vi "Main Page.vi"(8 "error in (no error)":errorcluster, 11 "Node Ptr":T5 format="%.0x") -> (0 "error out":errorcluster)   [LabVIEW 2017, in "ALMA_10201-10401_O2SensorSim System Explorer.lvlib"]
uses:
  ALMA_10201-10401_O2SensorSim System Explorer.lvlib
  Engine/LambdaType.ctl
  <vilib>/NI Veristand/Custom Device API/Custom Device Item Ref.ctl
  Engine/Par.ctl
  <vilib>/Utility/sysdir.llb/System Directory Type.ctl
  Shared/Constants.vi
  <vilib>/NI Veristand/Custom Device API/Get Item Property (U32).vi
  <vilib>/NI Veristand/Custom Device API/Get Item Property (Boolean).vi
  <vilib>/NI Veristand/Custom Device API/Set Item Property (Boolean).vi
  <vilib>/NI Veristand/Custom Device API/Get Item Property (String).vi
  <userlib>/_OpenG.lib/comparison/comparison.llb/I32 Changed__ogtk.vi
  <userlib>/_OpenG.lib/comparison/comparison.llb/Variant Changed__ogtk.vi
  <vilib>/NI Veristand/Custom Device API/Set Item Property (String).vi
  <vilib>/NI Veristand/Custom Device API/Custom Device API.lvlib
  <vilib>/NI Veristand/Custom Device API/Set Item Property (U32).vi
  Shared/ALMA_10201-10401_O2SensorSim Shared.lvlib
panel:
  out "product.Num":u32
  out "vendor.Num":u32
  out "SLSC Module Name":string
  out "Version":string
  out "Board":string
  out "Module Number":u32
  out "Temperature [°C] VS Rs [W]":cluster{"Custom Temp":dbl[], "Custom Ohm":dbl[]}(graph)
  out "l VS IP [mA]":T1(graph)
  in  "Mode":u16(ring) items=["SLSC Mode", "ANALOG Mode"]
  out "RefArray":refnum<vi>[](array[refnum])
  in  "Processor":i32=-2
  in  "Period [ms]":i64=100
  in  "Manual":bool
  in  "Description":string
  in  "Name":string
  in  "ParamUpdate":bool=TRUE
  in  "par 3":T2={"Loop time"={"Period [ms]"=0, "Processor"=0}, "COM"={"COM IP"="0.0.0.0", "COM port"=1, "Local port"=0, "Next_IP 1"=0, "Next_IP 2"=0, "Next_IP 3"=0, "Next_IP 4"=0}, "O2Sensor1"={"Lambda"={"LSU4.2 Lambda"=[], "LSU4.2 Ip"=[], "LSU4.9 Lambda"=[], "LSU4.9 Ip"=[], "LZA03 Lambda"=[], "LZA03 Ip"=[], "LZA08 Lambda"=[], "LZA08 Ip"=[], "Custom Lambda"=[], "Custom Ip"=[]}, "Temp"={"LSU4.2 Temp"=[], "LSU4.2 Ohm"=[], "LSU4.9 Temp"=[], "LSU4.9 Ohm"=[], "LZA03 Temp"=[], "LZA03 Ohm"=[], "LZA08 Temp"=[], "LZA08 Ohm"=[], "Custom Temp"=[], "Custom Ohm"=[]}, "Lambda Type"=0, "PID"={"Ki"=0.0, "Kp"=0.0, "Kd"=0.0, "FeedFW"=0.0}}, "O2Sensor2"={"Lambda"={"LSU4.2 Lambda"=[], "LSU4.2 Ip"=[], "LSU4.9 Lambda"=[], "LSU4.9 Ip"=[], "LZA03 Lambda"=[], "LZA03 Ip"=[], "LZA08 Lambda"=[], "LZA08 Ip"=[], "Custom Lambda"=[], "Custom Ip"=[]}, "Temp"={"LSU4.2 Temp"=[], "LSU4.2 Ohm"=[], "LSU4.9 Temp"=[], "LSU4.9 Ohm"=[], "LZA03 Temp"=[], "LZA03 Ohm"=[], "LZA08 Temp"=[], "LZA08 Ohm"=[], "Custom Temp"=[], "Custom Ohm"=[]}, "Lambda Type"=0, "PID"={"Ki"=0.0, "Kp"=0.0, "Kd"=0.0, "FeedFW"=0.0}}, "O2Sensor3"={"Lambda"={"LSU4.2 Lambda"=[], "LSU4.2 Ip"=[], "LSU4.9 Lambda"=[], "LSU4.9 Ip"=[], "LZA03 Lambda"=[], "LZA03 Ip"=[], "LZA08 Lambda"=[], "LZA08 Ip"=[], "Custom Lambda"=[], "Custom Ip"=[]}, "Temp"={"LSU4.2 Temp"=[], "LSU4.2 Ohm"=[], "LSU4.9 Temp"=[], "LSU4.9 Ohm"=[], "LZA03 Temp"=[], "LZA03 Ohm"=[], "LZA08 Temp"=[], "LZA08 Ohm"=[], "Custom Temp"=[], "Custom Ohm"=[]}, "Lambda Type"=0, "PID"={"Ki"=0.0, "Kp"=0.0, "Kd"=0.0, "FeedFW"=0.0}}, "O2Sensor4"={"Lambda"={"LSU4.2 Lambda"=[], "LSU4.2 Ip"=[], "LSU4.9 Lambda"=[], "LSU4.9 Ip"=[], "LZA03 Lambda"=[], "LZA03 Ip"=[], "LZA08 Lambda"=[], "LZA08 Ip"=[], "Custom Lambda"=[], "Custom Ip"=[]}, "Temp"={"LSU4.2 Temp"=[], "LSU4.2 Ohm"=[], "LSU4.9 Temp"=[], "LSU4.9 Ohm"=[], "LZA03 Temp"=[], "LZA03 Ohm"=[], "LZA08 Temp"=[], "LZA08 Ohm"=[], "Custom Temp"=[], "Custom Ohm"=[]}, "Lambda Type"=0, "PID"={"Ki"=0.0, "Kp"=0.0, "Kd"=0.0, "FeedFW"=0.0}}, "#ch_choise"=enum."O2Sim_2ch", "Mode"=enum."SLSC Mode", "vendor.Num"=4141, "product.Num"=0} {"O2Sensor4"."Lambda Type" items=["LSU4.2", "LSU4.9", "LZA03", "LZA08", "Custom", "[mA]"]; "O2Sensor3"."Lambda Type" items=["LSU4.2", "LSU4.9", "LZA03", "LZA08", "Custom", "[mA]"]; "O2Sensor2"."Lambda Type" items=["LSU4.2", "LSU4.9", "LZA03", "LZA08", "Custom", "[mA]"]; "O2Sensor1"."Lambda Type" items=["LSU4.2", "LSU4.9", "LZA03", "LZA08", "Custom", "[mA]"]}
  in  "Tab Control 2":T4(tab)=enum."O2Sensor4"
  in  "Caratteristica LSU4.2":dbl[][](array[numeric])
  in  "Caratteristica Bosch":dbl[][](array[numeric])
  in  "Caratteristica LZA08":dbl[][](array[numeric])
  in  "Caratteristica LZA03":dbl[][](array[numeric])
  in  "Caratteristica Custom":dbl[][](array[numeric])
  in  "Caratteristica LSU4.2_temp":dbl[][](array[numeric])
  in  "Caratteristica Bosch_temp":dbl[][](array[numeric])
  in  "Caratteristica LZA03_temp":dbl[][](array[numeric])
  in  "Caratteristica LZA08_temp":dbl[][](array[numeric])
  in  "Caratteristica Custom_temp":dbl[][](array[numeric])
  in  "Lambda":string="Lambda"
  in  "Ip [mA]":string="Ip [mA]"
  in  "Temp [°]":string="Temp [°]"
  in  "R [Ohm]":string="R [Ohm]"
  in  "O2Sensor Type":T3 items=["LSU4.2", "LSU4.9", "LZA03", "LZA08", "Custom", "[mA]"]
  in  "PID.Kp_1":dbl
  in  "PID.Kd_1":dbl
  in  "PID.FeedFW_1":dbl
  in  "PID.Ki_1":dbl
  in  "Import":bool
  in  "Caratteristica Custom 2":dbl[][](array[numeric])
  in  "Caratteristica LZA03 2":dbl[][](array[numeric])
  in  "Caratteristica LZA08 2":dbl[][](array[numeric])
  in  "Caratteristica Bosch 2":dbl[][](array[numeric])
  in  "Caratteristica LSU4.2 2":dbl[][](array[numeric])
  in  "Caratteristica Custom_temp 2":dbl[][](array[numeric])
  in  "Caratteristica LZA08_temp 2":dbl[][](array[numeric])
  in  "Caratteristica LZA03_temp 2":dbl[][](array[numeric])
  in  "Caratteristica Bosch_temp 2":dbl[][](array[numeric])
  in  "Caratteristica LSU4.2_temp 2":dbl[][](array[numeric])
  in  "R [Ohm] 2":string="R [Ohm]"
  in  "Temp [°] 2":string="Temp [°]"
  in  "Ip [mA] 2":string="Ip [mA]"
  in  "Lambda 2":string="Lambda"
  in  "PID.Ki_2":dbl=0.005
  in  "PID.FeedFW_2":dbl
  in  "PID.Kd_2":dbl
  in  "PID.Kp_2":dbl=100.0
  in  "O2Sensor Type 2":T3 items=["LSU4.2", "LSU4.9", "LZA03", "LZA08", "Custom", "[mA]"]
  in  "Import 2":bool
  in  "Caratteristica Custom 3":dbl[][](array[numeric])
  in  "Caratteristica LZA03 3":dbl[][](array[numeric])
  in  "Caratteristica LZA08 3":dbl[][](array[numeric])
  in  "Caratteristica Bosch 3":dbl[][](array[numeric])
  in  "Caratteristica LSU4.2 3":dbl[][](array[numeric])
  in  "Caratteristica Custom_temp 3":dbl[][](array[numeric])
  in  "Caratteristica LZA08_temp 3":dbl[][](array[numeric])
  in  "Caratteristica LZA03_temp 3":dbl[][](array[numeric])
  in  "Caratteristica Bosch_temp 3":dbl[][](array[numeric])
  in  "Caratteristica LSU4.2_temp 3":dbl[][](array[numeric])
  in  "R [Ohm] 3":string="R [Ohm]"
  in  "Temp [°] 3":string="Temp [°]"
  in  "Ip [mA] 3":string="Ip [mA]"
  in  "Lambda 3":string="Lambda"
  in  "PID.Ki_3":dbl=0.005
  in  "PID.FeedFW_3":dbl
  in  "PID.Kd_3":dbl
  in  "PID.Kp_3":dbl=100.0
  in  "O2Sensor Type 3":T3 items=["LSU4.2", "LSU4.9", "LZA03", "LZA08", "Custom", "[mA]"]
  in  "Import 3":bool
  in  "Caratteristica LSU4.2 4":dbl[][](array[numeric])
  in  "Caratteristica Bosch 4":dbl[][](array[numeric])
  in  "Caratteristica LZA03 4":dbl[][](array[numeric])
  in  "Caratteristica LZA08 4":dbl[][](array[numeric])
  in  "Caratteristica Custom 4":dbl[][](array[numeric])
  in  "Caratteristica LSU4.2_temp 4":dbl[][](array[numeric])
  in  "Caratteristica Custom_temp 4":dbl[][](array[numeric])
  in  "Caratteristica LZA08_temp 4":dbl[][](array[numeric])
  in  "Caratteristica LZA03_temp 4":dbl[][](array[numeric])
  in  "Caratteristica Bosch_temp 4":dbl[][](array[numeric])
  in  "Temp [°] 4":string="Temp [°]"
  in  "Ip [mA] 4":string="Ip [mA]"
  in  "Lambda 4":string="Lambda"
  in  "PID.Ki_4":dbl=0.005
  in  "PID.Kd_4":dbl
  in  "PID.Kp_4":dbl=100.0
  in  "O2Sensor Type 4":T3 items=["LSU4.2", "LSU4.9", "LZA03", "LZA08", "Custom", "[mA]"]
  in  "Import 4":bool
  in  "PID.FeedFW_4":dbl
  in  "R [Ohm] 4":string="R [Ohm]"
  in  "Header":cluster{"Section Name":string}={"Section Name"="Custom Device Item Settings"}
  # "l VS IP [mA]_"
  # "Temperature [°C] VS Rs [W]_"
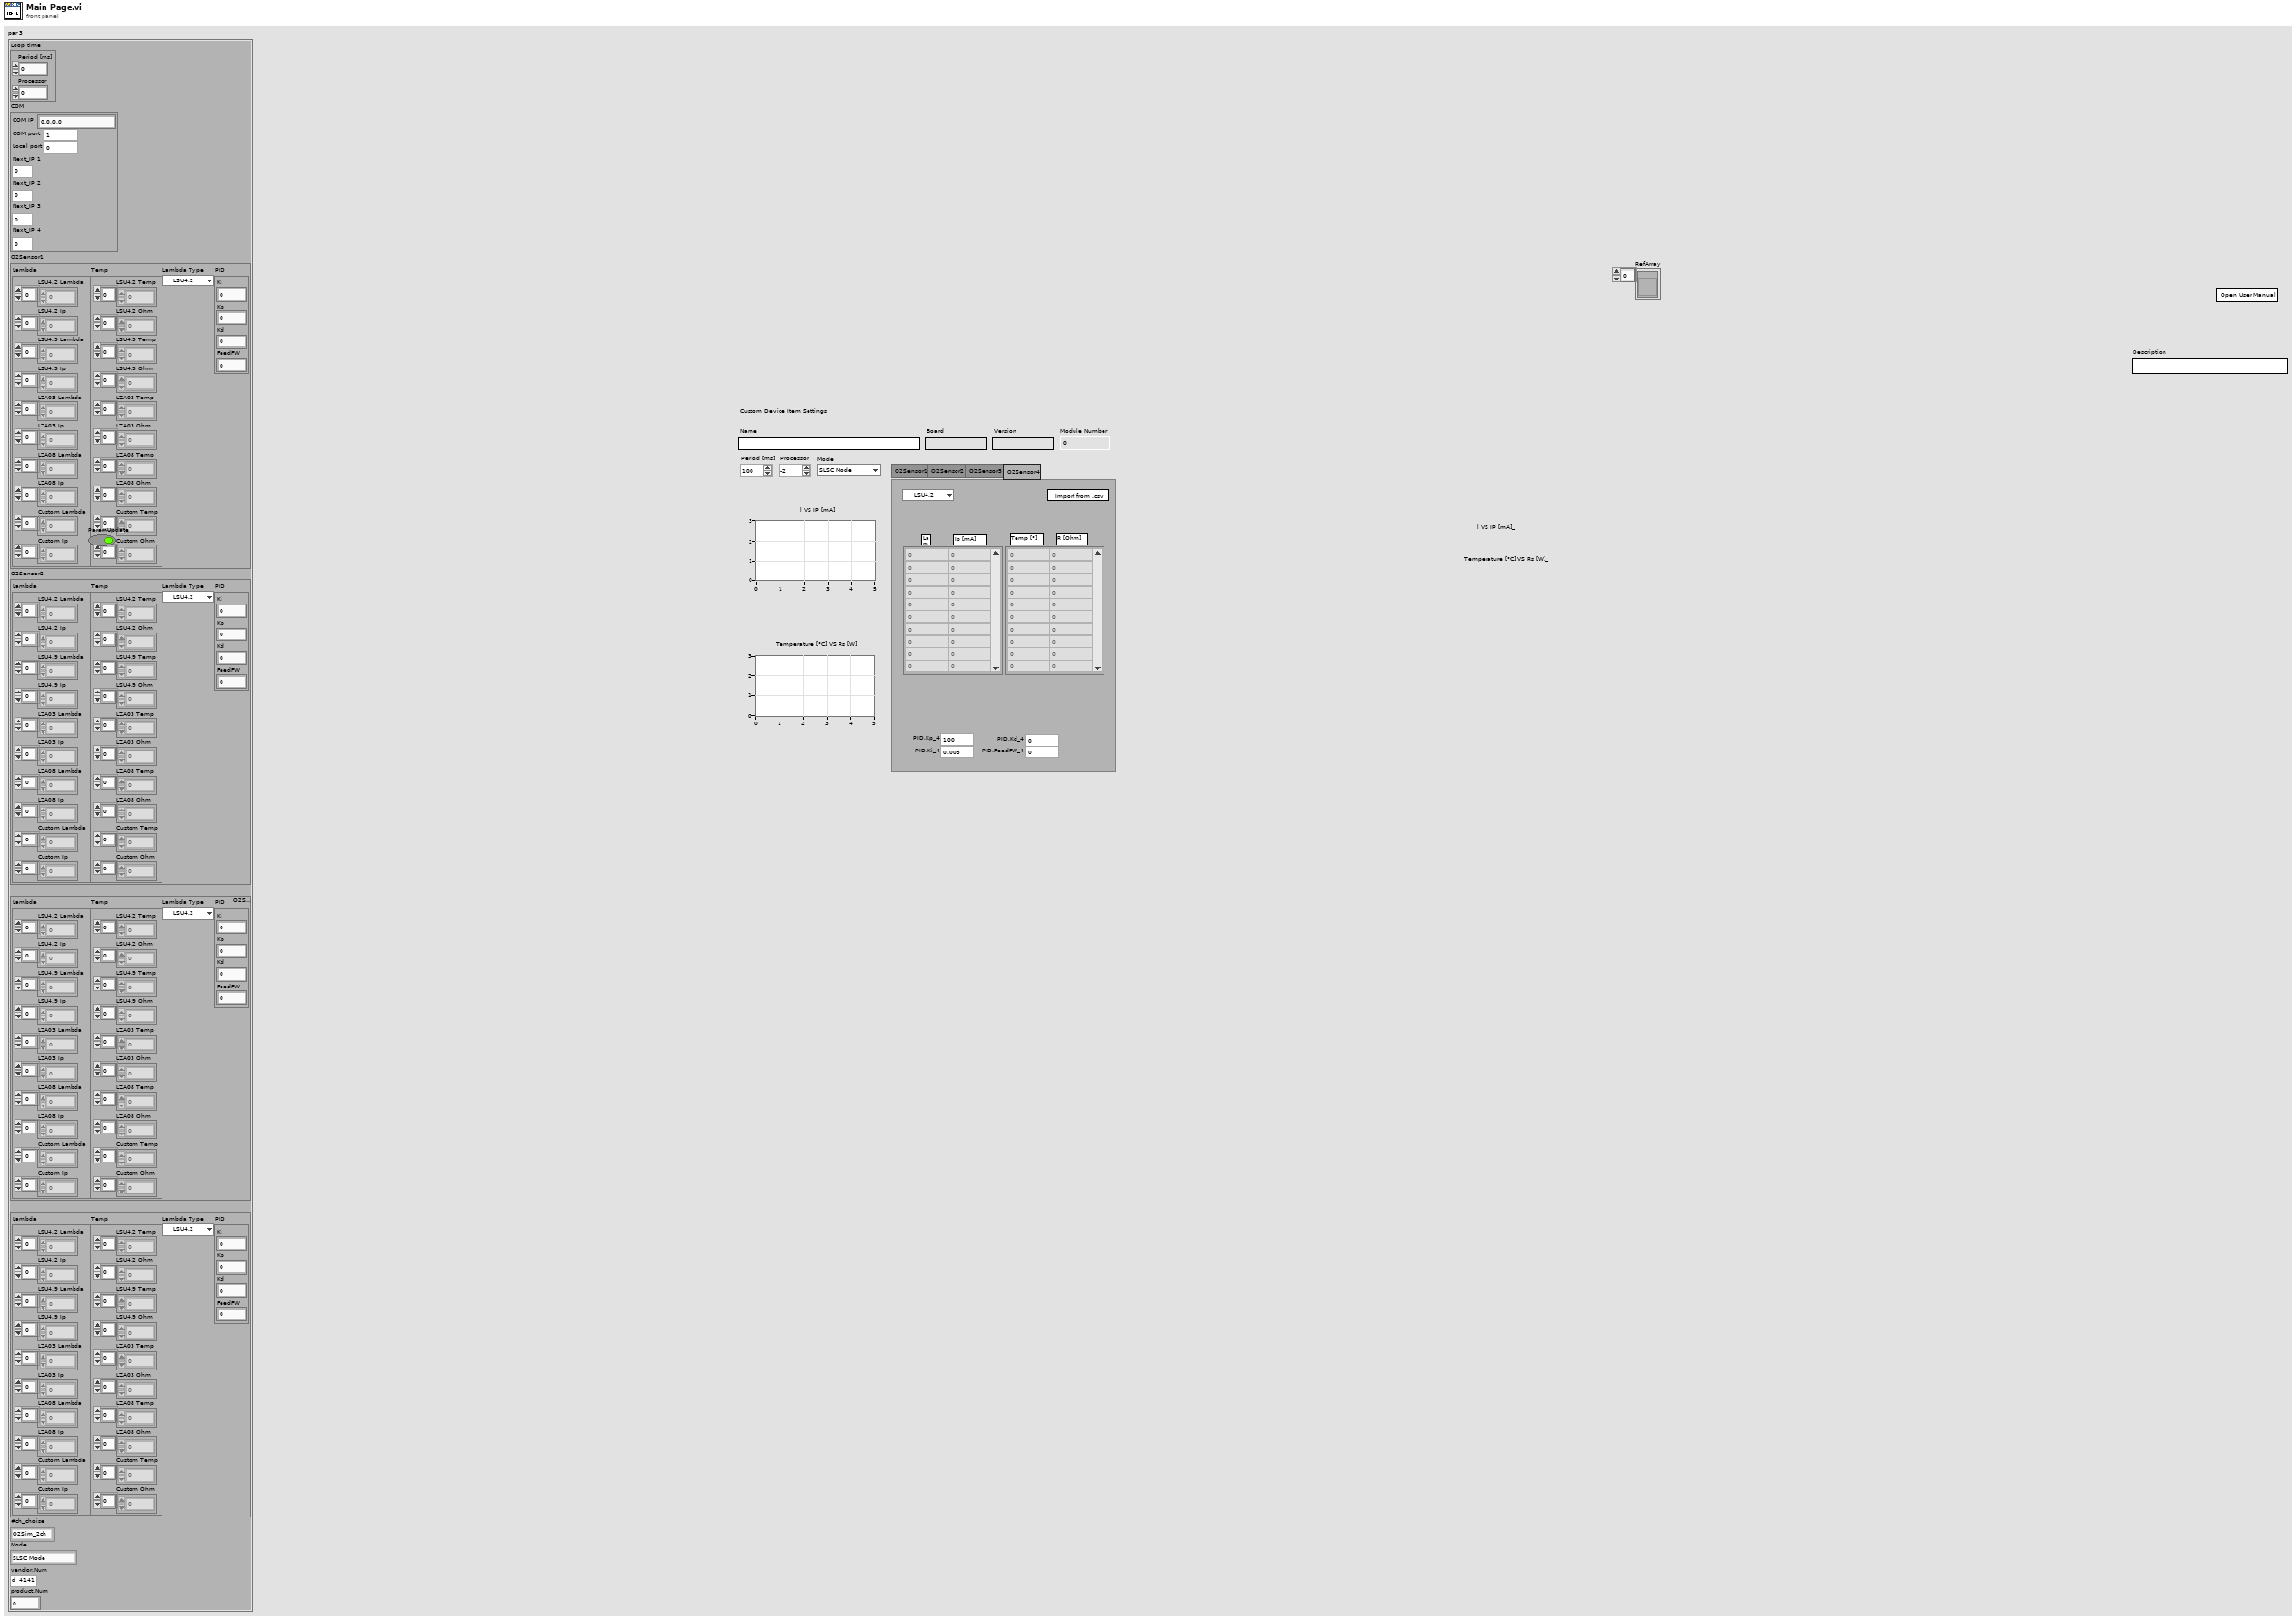
[diagram p1: front panel]
types:
  T1 = cluster{"Custom Lambda":dbl[], "Custom Ip":dbl[]}
  T2 = typedef "Par.ctl" = cluster{"Loop time":cluster{"Period [ms]":i64, "Processor":i32}, "COM":cluster{"COM IP":string, "COM port":u64, "Local port":u64, "Next_IP 1":u32, "Next_IP 2":u32, "Next_IP 3":u32, "Next_IP 4":u32}, "O2Sensor1":cluster{"Lambda":cluster{"LSU4.2 Lambda":dbl[], "LSU4.2 Ip":dbl[], "LSU4.9 Lambda":dbl[], "LSU4.9 Ip":dbl[], "LZA03 Lambda":dbl[], "LZA03 Ip":dbl[], "LZA08 Lambda":dbl[], "LZA08 Ip":dbl[], "Custom Lambda":dbl[], "Custom Ip":dbl[]}, "Temp":cluster{"LSU4.2 Temp":dbl[], "LSU4.2 Ohm":dbl[], "LSU4.9 Temp":dbl[], "LSU4.9 Ohm":dbl[], "LZA03 Temp":dbl[], "LZA03 Ohm":dbl[], "LZA08 Temp":dbl[], "LZA08 Ohm":dbl[], "Custom Temp":dbl[], "Custom Ohm":dbl[]}, "Lambda Type":T3, "PID":cluster{"Ki":dbl, "Kp":dbl, "Kd":dbl, "FeedFW":dbl}}, "O2Sensor2":cluster{"Lambda":cluster{"LSU4.2 Lambda":dbl[], "LSU4.2 Ip":dbl[], "LSU4.9 Lambda":dbl[], "LSU4.9 Ip":dbl[], "LZA03 Lambda":dbl[], "LZA03 Ip":dbl[], "LZA08 Lambda":dbl[], "LZA08 Ip":dbl[], "Custom Lambda":dbl[], "Custom Ip":dbl[]}, "Temp":cluster{"LSU4.2 Temp":dbl[], "LSU4.2 Ohm":dbl[], "LSU4.9 Temp":dbl[], "LSU4.9 Ohm":dbl[], "LZA03 Temp":dbl[], "LZA03 Ohm":dbl[], "LZA08 Temp":dbl[], "LZA08 Ohm":dbl[], "Custom Temp":dbl[], "Custom Ohm":dbl[]}, "Lambda Type":T3, "PID":cluster{"Ki":dbl, "Kp":dbl, "Kd":dbl, "FeedFW":dbl}}, "O2Sensor3":cluster{"Lambda":cluster{"LSU4.2 Lambda":dbl[], "LSU4.2 Ip":dbl[], "LSU4.9 Lambda":dbl[], "LSU4.9 Ip":dbl[], "LZA03 Lambda":dbl[], "LZA03 Ip":dbl[], "LZA08 Lambda":dbl[], "LZA08 Ip":dbl[], "Custom Lambda":dbl[], "Custom Ip":dbl[]}, "Temp":cluster{"LSU4.2 Temp":dbl[], "LSU4.2 Ohm":dbl[], "LSU4.9 Temp":dbl[], "LSU4.9 Ohm":dbl[], "LZA03 Temp":dbl[], "LZA03 Ohm":dbl[], "LZA08 Temp":dbl[], "LZA08 Ohm":dbl[], "Custom Temp":dbl[], "Custom Ohm":dbl[]}, "Lambda Type":T3, "PID":cluster{"Ki":dbl, "Kp":dbl, "Kd":dbl, "FeedFW":dbl}}, "O2Sensor4":cluster{"Lambda":cluster{"LSU4.2 Lambda":dbl[], "LSU4.2 Ip":dbl[], "LSU4.9 Lambda":dbl[], "LSU4.9 Ip":dbl[], "LZA03 Lambda":dbl[], "LZA03 Ip":dbl[], "LZA08 Lambda":dbl[], "LZA08 Ip":dbl[], "Custom Lambda":dbl[], "Custom Ip":dbl[]}, "Temp":cluster{"LSU4.2 Temp":dbl[], "LSU4.2 Ohm":dbl[], "LSU4.9 Temp":dbl[], "LSU4.9 Ohm":dbl[], "LZA03 Temp":dbl[], "LZA03 Ohm":dbl[], "LZA08 Temp":dbl[], "LZA08 Ohm":dbl[], "Custom Temp":dbl[], "Custom Ohm":dbl[]}, "Lambda Type":T3, "PID":cluster{"Ki":dbl, "Kp":dbl, "Kd":dbl, "FeedFW":dbl}}, "#ch_choise":enum16{"O2Sim_2ch", "O2Sim_4ch"}, "Mode":enum16{"SLSC Mode", "ANALOG Mode"}, "vendor.Num":u32, "product.Num":u32}
  T3 = typedef "LambdaType.ctl" = u16
  T4 = enum32{"O2Sensor1", "O2Sensor2", "O2Sensor3", "O2Sensor4"}
  T5 = typedef "Custom Device API.lvlib/Custom Device Item Ref.ctl" = u64
  T6 = typedef "Custom Device API.lvlib/Custom Device Item Info.ctl" = cluster{"Name":string, "Is Channel":bool, "GUID":string, "Is Waveform":bool}
  T7 = typedef "EDSjsonStructure.ctl" = cluster{"vendorNum":u32, "vendorName":string, "vendorPrefix":string, "productNum":u32, "productName":string, "capsVersion":string, "capsSpecVersion":u32, "capsSpecOldestCompatibleVersion":u32, "enums":T8[], "properties":T9[], "commands":T10[], "scales":T11[], "physicalChannels":T12[], "registerMap":cluster{"registers":T13[]}}
  T8 = typedef "enum.ctl" = cluster{"name":string, "description-en":string, "values":cluster{"name":string, "description-en":string, "value":i32}[]}
  T9 = typedef "property.ctl" = cluster{"name":string, "description-en":string, "documentation-en":string, "dataType":string, "bitfield":string, "access":string, "scale":string, "value":variant, "min":variant, "max":variant, "default value":variant}
  T10 = typedef "command.ctl" = cluster{"name":string, "description-en":string, "documentation-en":string, "startBitfield":string, "waitTimeInMs":i32, "doneBitfield":string, "doneInterrupt":string, "doneTimeoutInMs":i32, "value":variant}
  T11 = typedef "scale.ctl" = cluster{"name":string, "description-en":string, "m":dbl, "b":dbl, "forwardCoeffs":dbl[], "reverseCoeffs":dbl[], "coercion":string, "table":cluster{"scaled":dbl, "unscaled":dbl}[]}
  T12 = typedef "physicalChannel.ctl" = cluster{"name":string, "description-en":string, "commands":T10[], "properties":T9[]}
  T13 = typedef "register.ctl" = cluster{"name":string, "description-en":string, "access":string, "address":u32, "size":u32, "bitfields":cluster{"name":string, "description-en":string, "offset":u32, "size":u32, "signed":bool, "strobe":bool}[]}
  T14 = cluster{"Lambda":cluster{"LSU4.2 Lambda":dbl[], "LSU4.2 Ip":dbl[], "LSU4.9 Lambda":dbl[], "LSU4.9 Ip":dbl[], "LZA03 Lambda":dbl[], "LZA03 Ip":dbl[], "LZA08 Lambda":dbl[], "LZA08 Ip":dbl[], "Custom Lambda":dbl[], "Custom Ip":dbl[]}, "Temp":cluster{"LSU4.2 Temp":dbl[], "LSU4.2 Ohm":dbl[], "LSU4.9 Temp":dbl[], "LSU4.9 Ohm":dbl[], "LZA03 Temp":dbl[], "LZA03 Ohm":dbl[], "LZA08 Temp":dbl[], "LZA08 Ohm":dbl[], "Custom Temp":dbl[], "Custom Ohm":dbl[]}, "Lambda Type":T3, "PID":cluster{"Ki":dbl, "Kp":dbl, "Kd":dbl, "FeedFW":dbl}}
  T15 = cluster{"Lambda":cluster{"LSU4.2 Lambda":dbl[], "LSU4.2 Ip":dbl[], "LSU4.9 Lambda":dbl[], "LSU4.9 Ip":dbl[], "LZA03 Lambda":dbl[], "LZA03 Ip":dbl[], "LZA08 Lambda":dbl[], "LZA08 Ip":dbl[], "Custom Lambda":dbl[], "Custom Ip":dbl[]}, "Temp":cluster{"LSU4.2 Temp":dbl[], "LSU4.2 Ohm":dbl[], "LSU4.9 Temp":dbl[], "LSU4.9 Ohm":dbl[], "LZA03 Temp":dbl[], "LZA03 Ohm":dbl[], "LZA08 Temp":dbl[], "LZA08 Ohm":dbl[], "Custom Temp":dbl[], "Custom Ohm":dbl[]}, "Lambda Type":T3, "PID":cluster{"Ki":dbl, "Kp":dbl, "Kd":dbl, "FeedFW":dbl}}[]
  T16 = enum16{"open", "replace", "create", "open or create", "replace or create", "replace or create with confirmation"}
  T17 = typedef "Custom Device API.lvlib/Custom Device Commands.ctl" = enum16{"Default", "Item renamed", "Shutdown", "Dynamic button pressed"}
  T18 = typedef "System Directory Type.ctl" = i32
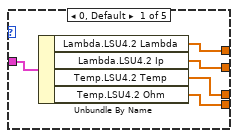
[diagram p4: hidden frame]
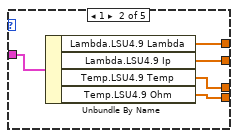
[diagram p5: hidden frame]
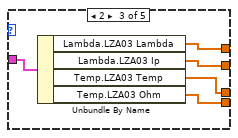
[diagram p6: hidden frame]
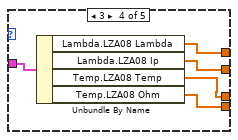
[diagram p7: hidden frame]
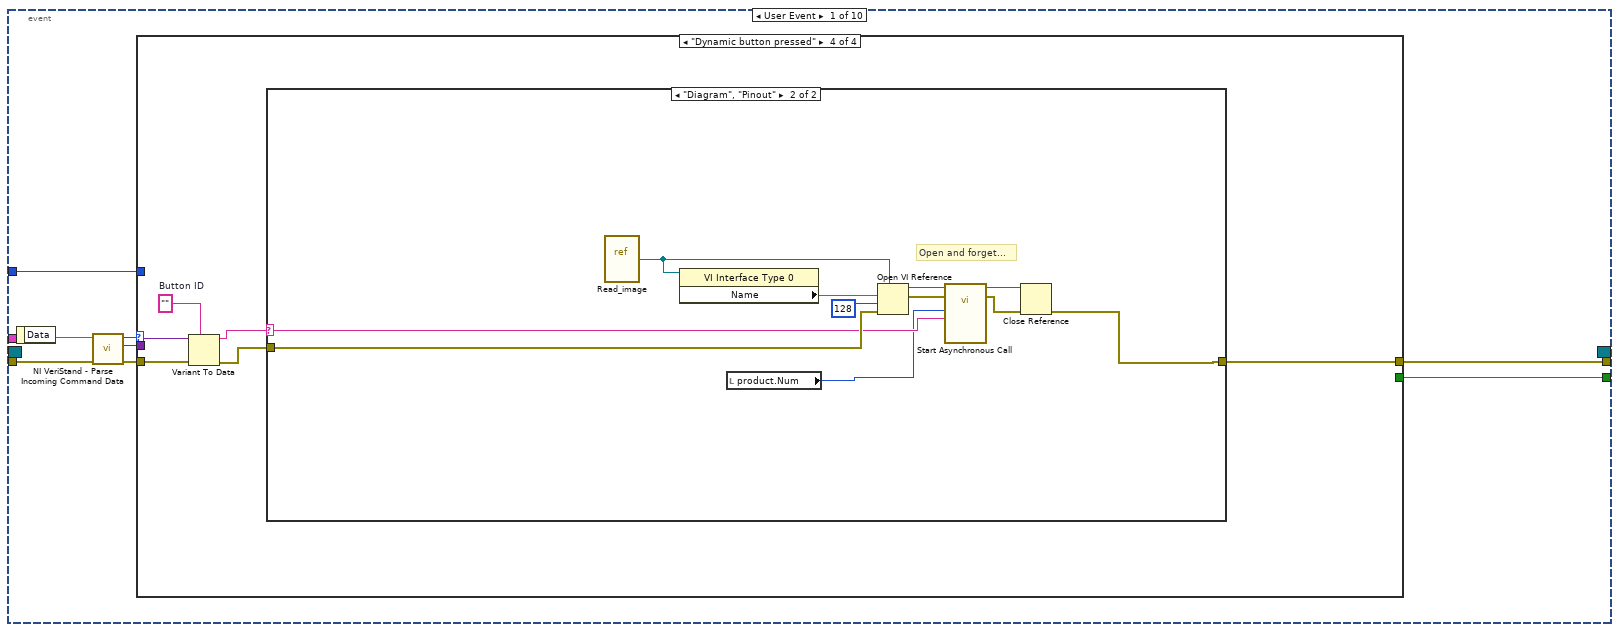
[diagram p9: hidden frame]
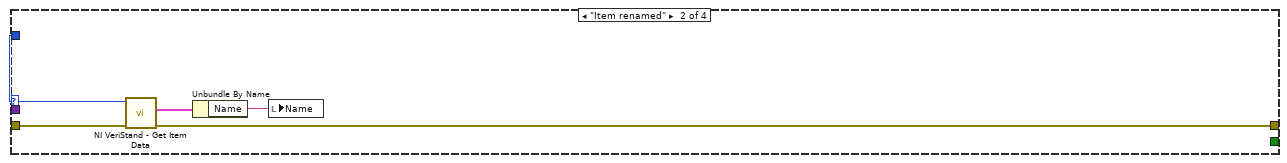
[diagram p11: hidden frame]
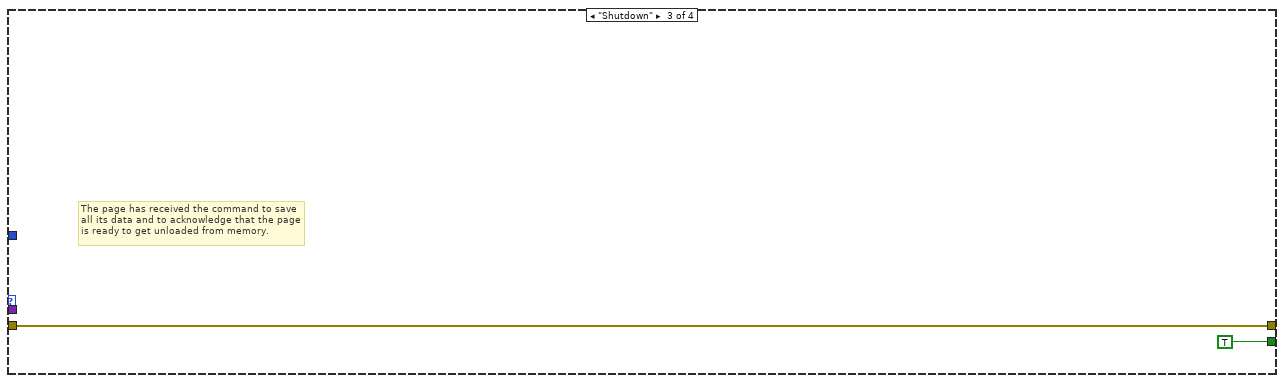
[diagram p12: hidden frame]
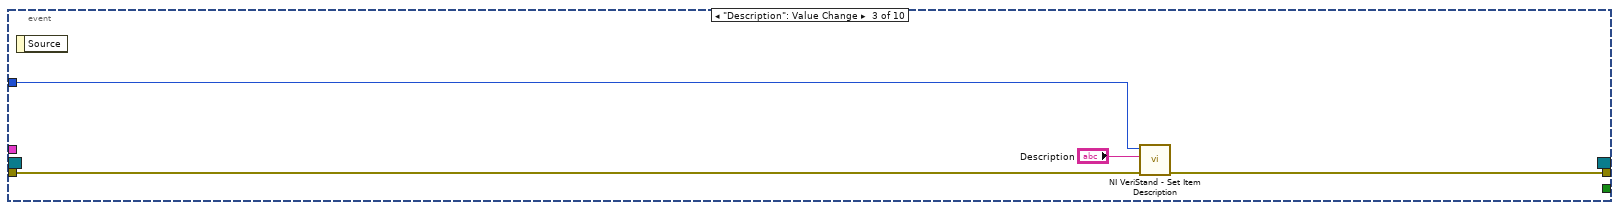
[diagram p14: hidden frame]
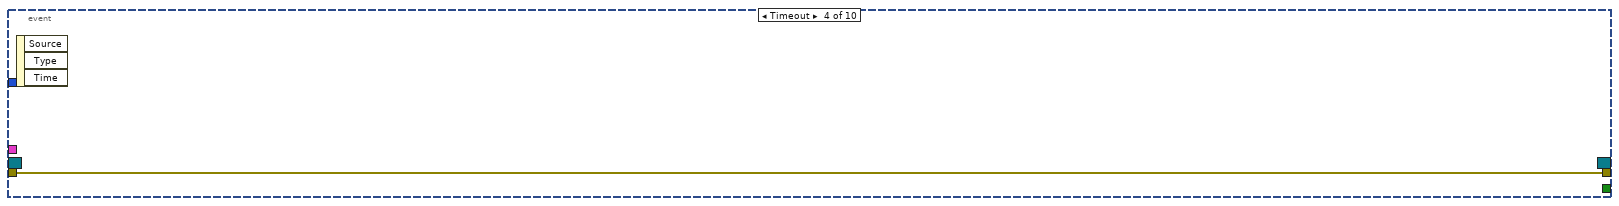
[diagram p15: hidden frame]
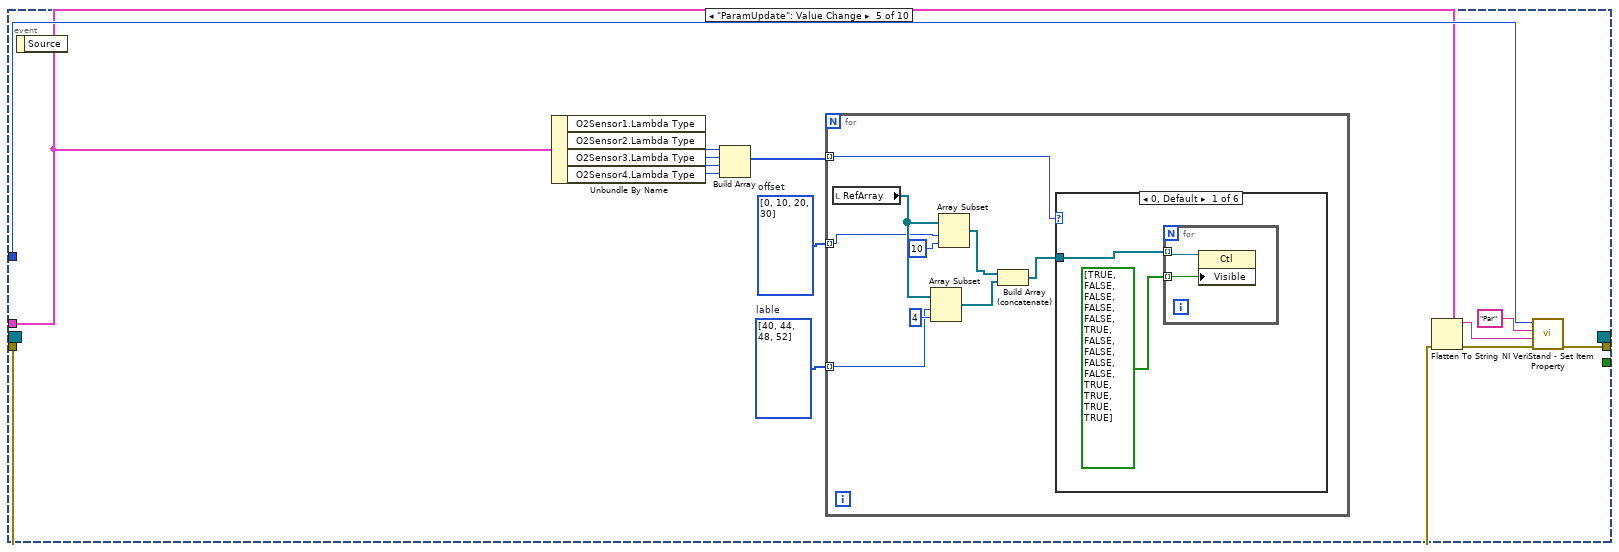
[diagram p16: hidden frame]
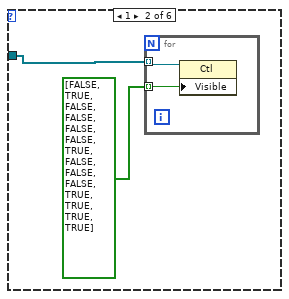
[diagram p17: hidden frame]
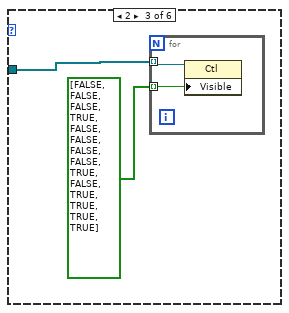
[diagram p18: hidden frame]
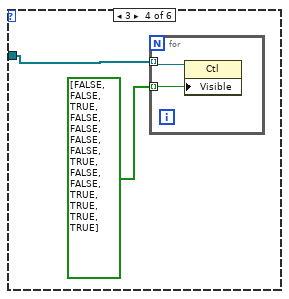
[diagram p19: hidden frame]
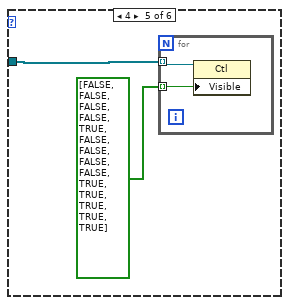
[diagram p20: hidden frame]
diagram:
  n1 = flat-sequence "Initialization code" {
    tunnel: "Node Ptr" -> [w15]
    tunnel: "error in (no error)" -> [w16]
    tunnel: [w16] -> w4
    tunnel: [w15] -> w3
    tunnel: [w100] -> w8
    tunnel: [w99] -> w6
    tunnel: w4 -> [w100]
    tunnel: w3 -> [w99]
    tunnel: w8 -> [w240]
    tunnel: [w240] -> w7
    tunnel: w6 -> [w239]
    tunnel: [w239] -> w5
    tunnel: w7 -> [w304]
    tunnel: w5 -> [w303]
    tunnel: [w308] -> w12
    tunnel: [w307] -> w2
    tunnel: [w306] -> w1
    frame #0 {
      # "52"
      # "48"
      # "44"
      # "40"
      # "35"
      # "30"
      # "25"
      # "20"
      # "15"
      # "10"
      # "5"
      # "0"
    }
    frame #1 {
      # "76"
      # "72"
      # "68"
      # "64"
      # "60"
      # "56"
      n2 = control-ref of="Import"() -> (w36:refnum<vi>)
      n3 = control-ref of="Import 2"() -> (w35:refnum<vi>)
      n4 = control-ref of="Import 3"() -> (w34:refnum<vi>)
      n5 = control-ref of="Import 4"() -> (w33:refnum<vi>)
      n6 = control-ref of="PID.Ki_1"() -> (w32:refnum<vi>)
      n7 = control-ref of="PID.Kp_1"() -> (w31:refnum<vi>)
      n8 = control-ref of="PID.Kd_1"() -> (w30:refnum<vi>)
      n9 = control-ref of="PID.FeedFW_1"() -> (w29:refnum<vi>)
      n10 = control-ref of="PID.Ki_2"() -> (w28:refnum<vi>)
      n11 = control-ref of="PID.Kp_2"() -> (w27:refnum<vi>)
      n12 = control-ref of="PID.Kd_2"() -> (w26:refnum<vi>)
      n13 = control-ref of="PID.FeedFW_2"() -> (w25:refnum<vi>)
      n14 = control-ref of="PID.Ki_3"() -> (w24:refnum<vi>)
      n15 = control-ref of="PID.Kp_3"() -> (w23:refnum<vi>)
      n16 = control-ref of="PID.Kd_3"() -> (w22:refnum<vi>)
      n17 = control-ref of="PID.FeedFW_3"() -> (w21:refnum<vi>)
      n18 = control-ref of="PID.Ki_4"() -> (w20:refnum<vi>)
      n19 = control-ref of="PID.Kp_4"() -> (w19:refnum<vi>)
      n20 = control-ref of="PID.Kd_4"() -> (w18:refnum<vi>)
      n21 = control-ref of="PID.FeedFW_4"() -> (w17:refnum<vi>)
      n22 = control-ref of="Caratteristica LSU4.2_temp 2"() -> (w83:refnum<vi>)
      n23 = control-ref of="Caratteristica Bosch_temp 2"() -> (w82:refnum<vi>)
      n24 = control-ref of="Caratteristica LZA03_temp 2"() -> (w81:refnum<vi>)
      n25 = control-ref of="Caratteristica LZA08_temp 2"() -> (w80:refnum<vi>)
      n26 = control-ref of="Caratteristica Custom_temp 2"() -> (w79:refnum<vi>)
      n27 = control-ref of="Caratteristica LSU4.2 2"() -> (w88:refnum<vi>)
      n28 = control-ref of="Caratteristica Bosch 2"() -> (w87:refnum<vi>)
      n29 = control-ref of="Caratteristica LZA08 2"() -> (w86:refnum<vi>)
      n30 = control-ref of="Caratteristica LZA03 2"() -> (w85:refnum<vi>)
      n31 = control-ref of="Caratteristica Custom 2"() -> (w84:refnum<vi>)
      n32 = control-ref of="Caratteristica LSU4.2 4"() -> (w68:refnum<vi>)
      n33 = control-ref of="Caratteristica Bosch 4"() -> (w67:refnum<vi>)
      n34 = control-ref of="Caratteristica LZA03 4"() -> (w66:refnum<vi>)
      n35 = control-ref of="Caratteristica LZA08 4"() -> (w65:refnum<vi>)
      n36 = control-ref of="Caratteristica Custom 4"() -> (w64:refnum<vi>)
      n37 = control-ref of="Caratteristica LSU4.2_temp 4"() -> (w63:refnum<vi>)
      n38 = control-ref of="Caratteristica Bosch_temp 4"() -> (w62:refnum<vi>)
      n39 = control-ref of="Caratteristica LZA03_temp 4"() -> (w61:refnum<vi>)
      n40 = control-ref of="Caratteristica LZA08_temp 4"() -> (w60:refnum<vi>)
      n41 = control-ref of="Caratteristica Custom_temp 4"() -> (w59:refnum<vi>)
      n42 = control-ref of="Caratteristica LSU4.2 3"() -> (w78:refnum<vi>)
      n43 = control-ref of="Caratteristica Bosch 3"() -> (w77:refnum<vi>)
      n44 = control-ref of="Caratteristica LZA08 3"() -> (w76:refnum<vi>)
      n45 = control-ref of="Caratteristica LZA03 3"() -> (w75:refnum<vi>)
      n46 = control-ref of="Caratteristica Custom 3"() -> (w74:refnum<vi>)
      n47 = control-ref of="Caratteristica LSU4.2_temp 3"() -> (w73:refnum<vi>)
      n48 = control-ref of="Caratteristica Bosch_temp 3"() -> (w72:refnum<vi>)
      n49 = control-ref of="Caratteristica LZA03_temp 3"() -> (w71:refnum<vi>)
      n50 = control-ref of="Caratteristica LZA08_temp 3"() -> (w70:refnum<vi>)
      n51 = control-ref of="Caratteristica Custom_temp 3"() -> (w69:refnum<vi>)
      n52 = control-ref of="Lambda"() -> (w58:refnum<vi>)
      n53 = control-ref of="Ip [mA]"() -> (w57:refnum<vi>)
      n54 = control-ref of="Temp [°]"() -> (w56:refnum<vi>)
      n55 = control-ref of="R [Ohm]"() -> (w55:refnum<vi>)
      n56 = control-ref of="Lambda 2"() -> (w54:refnum<vi>)
      n57 = control-ref of="Ip [mA] 2"() -> (w53:refnum<vi>)
      n58 = control-ref of="Temp [°] 2"() -> (w52:refnum<vi>)
      n59 = control-ref of="R [Ohm] 2"() -> (w51:refnum<vi>)
      n60 = control-ref of="Lambda 3"() -> (w50:refnum<vi>)
      n61 = control-ref of="Ip [mA] 3"() -> (w49:refnum<vi>)
      n62 = control-ref of="Temp [°] 3"() -> (w48:refnum<vi>)
      n63 = control-ref of="R [Ohm] 3"() -> (w47:refnum<vi>)
      n64 = control-ref of="Lambda 4"() -> (w46:refnum<vi>)
      n65 = control-ref of="Ip [mA] 4"() -> (w45:refnum<vi>)
      n66 = control-ref of="Temp [°] 4"() -> (w44:refnum<vi>)
      n67 = control-ref of="R [Ohm] 4"() -> (w43:refnum<vi>)
      n68 = control-ref of="O2Sensor Type"() -> (w40:refnum<vi>)
      n69 = control-ref of="O2Sensor Type 2"() -> (w39:refnum<vi>)
      n70 = control-ref of="O2Sensor Type 3"() -> (w38:refnum<vi>)
      n71 = control-ref of="O2Sensor Type 4"() -> (w37:refnum<vi>)
      n72 = control-ref of="Caratteristica LSU4.2_temp"() -> (w93:refnum<vi>)
      n73 = control-ref of="Caratteristica Bosch_temp"() -> (w92:refnum<vi>)
      n74 = control-ref of="Caratteristica LZA03_temp"() -> (w91:refnum<vi>)
      n75 = control-ref of="Caratteristica LZA08_temp"() -> (w90:refnum<vi>)
      n76 = control-ref of="Caratteristica Custom_temp"() -> (w89:refnum<vi>)
      n77 = control-ref of="Caratteristica LSU4.2"() -> (w98:refnum<vi>)
      n78 = control-ref of="Caratteristica Bosch"() -> (w97:refnum<vi>)
      n79 = control-ref of="Caratteristica LZA08"() -> (w96:refnum<vi>)
      n80 = control-ref of="Caratteristica LZA03"() -> (w95:refnum<vi>)
      n81 = control-ref of="Caratteristica Custom"() -> (w94:refnum<vi>)
      n82 = Build Array(w40, w39, w38, w37, w36, w35, w34, w33, w32, w31, w30, w29, w28, w27, w26, w25, w24, w23, w22, w21, w20, w19, w18, w17) -> (w41:refnum<vi>[])
      n83 = Build Array (concatenate)(w98, w97, w96, w95, w94, w93, w92, w91, w90, w89, w88, w87, w86, w85, w84, w83, w82, w81, w80, w79, w78, w77, w76, w75, w74, w73, w72, w71, w70, w69, w68, w67, w66, w65, w64, w63, w62, w61, w60, w59, w58, w57, w56, w55, w54, w53, w52, w51, w50, w49, w48, w47, w46, w45, w44, w43, w41) -> (→"RefArray":refnum<vi>[])
    }
    frame #2 {
      n84 = local read "RefArray"() -> (w101:refnum<vi>[])
      n85 = Index Array(array=w101) -> (element=w226:refnum<vi>)  [unwired: 1 in]
      n86 = Index Array(array=w101, index #1=40 ("index"), index #2=44 ("index"), index #3=48 ("index"), index #4=52 ("index")) -> (element #1=w205:refnum<vi>, element #2=w197:refnum<vi>, element #3=w196:refnum<vi>, element #4=w195:refnum<vi>)
      n87 = Index Array(array=w101, index=5) -> (element=w206:refnum<vi>)
      n88 = Index Array(array=w101, index #1=41 ("index"), index #2=45 ("index"), index #3=49 ("index"), index #4=53 ("index")) -> (element #1=w184:refnum<vi>, element #2=w192:refnum<vi>, element #3=w193:refnum<vi>, element #4=w194:refnum<vi>)
      n89 = Index Array(array=w101, index #1=56 ("index")) -> (element #1=w161:refnum<vi>, element #2=w156:refnum<vi>, element #3=w155:refnum<vi>, element #4=w154:refnum<vi>)  [unwired: 3 in]
      n90 = Index Array(array=w101, index #1=42 ("index"), index #2=46 ("index"), index #3=50 ("index"), index #4=54 ("index")) -> (element #1=w183:refnum<vi>, element #2=w175:refnum<vi>, element #3=w174:refnum<vi>, element #4=w173:refnum<vi>)
      n91 = Index Array(array=w101, index #1=43 ("index"), index #2=47 ("index"), index #3=51 ("index"), index #4=55 ("index")) -> (element #1=w162:refnum<vi>, element #2=w170:refnum<vi>, element #3=w171:refnum<vi>, element #4=w172:refnum<vi>)
      n92 = Index Array(array=w101, index #1=60 ("index")) -> (element #1=w146:refnum<vi>, element #2=w151:refnum<vi>, element #3=w152:refnum<vi>, element #4=w153:refnum<vi>)  [unwired: 3 in]
      n93 = Index Array(array=w101, index #1=64 ("index"), index #2=68 ("index"), index #3=72 ("index"), index #4=76 ("index")) -> (element #1=w102:refnum<vi>, element #2=w110:refnum<vi>, element #3=w111:refnum<vi>, element #4=w112:refnum<vi>)
      n94 = Index Array(array=w101, index #1=65 ("index"), index #2=69 ("index"), index #3=73 ("index"), index #4=77 ("index")) -> (element #1=w123:refnum<vi>, element #2=w115:refnum<vi>, element #3=w114:refnum<vi>, element #4=w113:refnum<vi>)
      n95 = Array Subset(array=w101, index=35, length=5) -> (w232:refnum<vi>[])
      n96 = Index Array(array=w101, index #1=66 ("index"), index #2=70 ("index"), index #3=74 ("index"), index #4=78 ("index")) -> (element #1=w124:refnum<vi>, element #2=w132:refnum<vi>, element #3=w133:refnum<vi>, element #4=w134:refnum<vi>)
      n97 = Array Subset(array=w101, index=25, length=5) -> (w233:refnum<vi>[])
      n98 = Index Array(array=w101, index #1=67 ("index"), index #2=71 ("index"), index #3=75 ("index"), index #4=79 ("index")) -> (element #1=w145:refnum<vi>, element #2=w137:refnum<vi>, element #3=w136:refnum<vi>, element #4=w135:refnum<vi>)
      n99 = Array Subset(array=w101, index=6, length=4) -> (w234:refnum<vi>[])
      n100 = Array Subset(array=w101, index=15, length=5) -> (w235:refnum<vi>[])
      n101 = Array Subset(array=w101, index=30, length=5) -> (w231:refnum<vi>[])
      n102 = Array Subset(array=w101, index=20, length=5) -> (w230:refnum<vi>[])
      n103 = Array Subset(array=w101, index=1, length=4) -> (w225:refnum<vi>[])
      n104 = Array Subset(array=w101, index=10, length=5) -> (w224:refnum<vi>[])
      n105 = property class="Ctl"(reference=w226) -> ("Left"=w228:i32, "Top"=w229:i32)  [unwired: 1 in, 2 out]
      n106 = property class="Ctl"(reference=w206) -> ("Left"=w236:i32, "Top"=w237:i32)  [unwired: 1 in, 2 out]
      n107 = property class="Ctl"(reference=w205) -> ("Left"=w203:i32, "Top"=w202:i32)  [unwired: 1 in, 2 out]
      n108 = property class="Ctl"(reference=w184) -> ("Left"=w186:i32, "Top"=w187:i32)  [unwired: 1 in, 2 out]
      n109 = property class="Ctl"(reference=w161) -> ("Left"=w159:i32, "Top"=w158:i32)  [unwired: 1 in, 2 out]
      n110 = property class="Ctl"(reference=w183) -> ("Left"=w181:i32, "Top"=w180:i32)  [unwired: 1 in, 2 out]
      n111 = property class="Ctl"(reference=w162) -> ("Left"=w164:i32, "Top"=w165:i32)  [unwired: 1 in, 2 out]
      n112 = property class="Ctl"(reference=w146) -> ("Left"=w148:i32, "Top"=w149:i32)  [unwired: 1 in, 2 out]
      n113 = property class="Ctl"(reference=w102) -> ("Left"=w104:i32, "Top"=w105:i32)  [unwired: 1 in, 2 out]
      n114 = property class="Ctl"(reference=w123) -> ("Left"=w121:i32, "Top"=w120:i32)  [unwired: 1 in, 2 out]
      n115 = Build Array (concatenate)(w234, w235, w233, w232) -> (w238:refnum<vi>[])
      n116 = property class="Ctl"(reference=w124) -> ("Left"=w126:i32, "Top"=w127:i32)  [unwired: 1 in, 2 out]
      n117 = property class="Ctl"(reference=w145) -> ("Left"=w143:i32, "Top"=w142:i32)  [unwired: 1 in, 2 out]
      n118 = Build Array(w197, w196, w195) -> (w201:refnum<vi>[])
      n119 = Build Array(w192, w193, w194) -> (w188:refnum<vi>[])
      n120 = Build Array (concatenate)(w225, w224, w230, w231) -> (w227:refnum<vi>[])
      n121 = Build Array(w156, w155, w154) -> (w157:refnum<vi>[])
      n122 = Build Array(w175, w174, w173) -> (w179:refnum<vi>[])
      n123 = Build Array(w170, w171, w172) -> (w166:refnum<vi>[])
      n124 = Build Array(w151, w152, w153) -> (w150:refnum<vi>[])
      n125 = Build Array(w110, w111, w112) -> (w106:refnum<vi>[])
      n126 = Build Array(w115, w114, w113) -> (w119:refnum<vi>[])
      n127 = Build Array(w132, w133, w134) -> (w128:refnum<vi>[])
      n128 = Build Array(w137, w136, w135) -> (w141:refnum<vi>[])
      n129 = for {
        tunnel: w238 -> [w273] mode=indexing
        tunnel: w236 -> [w272]
        tunnel: w237 -> [w271]
        n130 = property class="Ctl"(reference=w273, "Left"=w272, "Top"=w271) -> ()  [unwired: 1 in, 2 out]
      }
      n131 = for {
        tunnel: w201 -> [w270] mode=indexing
        tunnel: w203 -> [w269]
        tunnel: w202 -> [w268]
        n132 = property class="Ctl"(reference=w270, "Left"=w269, "Top"=w268) -> ()  [unwired: 1 in, 2 out]
      }
      n133 = for {
        tunnel: w188 -> [w267] mode=indexing
        tunnel: w186 -> [w266]
        tunnel: w187 -> [w265]
        n134 = property class="Ctl"(reference=w267, "Left"=w266, "Top"=w265) -> ()  [unwired: 1 in, 2 out]
      }
      n135 = for {
        tunnel: w157 -> [w258] mode=indexing
        tunnel: w159 -> [w257]
        tunnel: w158 -> [w256]
        n136 = property class="Ctl"(reference=w258, "Left"=w257, "Top"=w256) -> ()  [unwired: 1 in, 2 out]
      }
      n137 = for {
        tunnel: w179 -> [w264] mode=indexing
        tunnel: w181 -> [w263]
        tunnel: w180 -> [w262]
        n138 = property class="Ctl"(reference=w264, "Left"=w263, "Top"=w262) -> ()  [unwired: 1 in, 2 out]
      }
      n139 = for {
        tunnel: w166 -> [w261] mode=indexing
        tunnel: w164 -> [w260]
        tunnel: w165 -> [w259]
        n140 = property class="Ctl"(reference=w261, "Left"=w260, "Top"=w259) -> ()  [unwired: 1 in, 2 out]
      }
      n141 = for {
        tunnel: w150 -> [w255] mode=indexing
        tunnel: w148 -> [w254]
        tunnel: w149 -> [w253]
        n142 = property class="Ctl"(reference=w255, "Left"=w254, "Top"=w253) -> ()  [unwired: 1 in, 2 out]
      }
      n143 = for {
        tunnel: w227 -> [w276] mode=indexing
        tunnel: w228 -> [w275]
        tunnel: w229 -> [w274]
        n144 = property class="Ctl"(reference=w276, "Left"=w275, "Top"=w274) -> ()  [unwired: 1 in, 2 out]
      }
      n145 = for {
        tunnel: w106 -> [w252] mode=indexing
        tunnel: w104 -> [w251]
        tunnel: w105 -> [w250]
        n146 = property class="Ctl"(reference=w252, "Left"=w251, "Top"=w250) -> ()  [unwired: 1 in, 2 out]
      }
      n147 = for {
        tunnel: w119 -> [w249] mode=indexing
        tunnel: w121 -> [w248]
        tunnel: w120 -> [w247]
        n148 = property class="Ctl"(reference=w249, "Left"=w248, "Top"=w247) -> ()  [unwired: 1 in, 2 out]
      }
      n149 = for {
        tunnel: w128 -> [w246] mode=indexing
        tunnel: w126 -> [w245]
        tunnel: w127 -> [w244]
        n150 = property class="Ctl"(reference=w246, "Left"=w245, "Top"=w244) -> ()  [unwired: 1 in, 2 out]
      }
      n151 = for {
        tunnel: w141 -> [w243] mode=indexing
        tunnel: w143 -> [w242]
        tunnel: w142 -> [w241]
        n152 = property class="Ctl"(reference=w243, "Left"=w242, "Top"=w241) -> ()  [unwired: 1 in, 2 out]
      }
    }
    frame #3 {
      w310 = i32[] [40, 44, 48, 52]  # lable
      w313 = i32[] [0, 10, 20, 30]  # offset
      w311 = i32[] [64, 68, 72, 76]  # PID
      w312 = i32[] [56, 57, 58, 59]  # lambda type
      n153 = call <vilib>:"NI VeriStand - Get Item Description.vi"("error in (no error)"=w304, "Item Ref in"=w303) -> ("error out"=w325:errorcluster, "Description"=w326:string, "Item Ref out"=w327:T5)  [unwired: 7 out]
      n154 = local write "Description"(w326) -> ()
      n155 = call <vilib>:"NI VeriStand - Get Item Data.vi"("error in (no error)"=w325, "Item Ref in"=w327) -> ("error out"=w298:errorcluster, "Item Info"=w324:T6, "Item Ref out"=w299:T5)  [unwired: 7 out]
      n156 = Unbundle By Name(w324) -> ("Name"=w320:string)
      n157 = local write "Name"(w320) -> ()
      n158 = call <vilib>:"NI VeriStand - Get Custom Device Version.vi"("error in (no error)"=w298, "Device Ref in"=w299) -> ("error out"=w286:errorcluster, "Value"=→"Version":string, "Device Ref out"=w285:T5)  [unwired: 7 in]
      n159 = global read "Constants.vi" "Module Number"() -> (w305:string)
      n160 = global read "Constants.vi" "initialized?"() -> (w295:string)
      n161 = call-poly <vilib>:"NI VeriStand - Get Item Property.vi"("error in (no error)"=w286, "Property Name"=w305, "Item Ref in"=w285) -> ("error out"=w292:errorcluster, "Value"=w289:u32, "Item Ref out"=w294:T5)  [unwired: 5 in, 1 out]
      "Module Number" <- w289
      n162 = call-poly <vilib>:"NI VeriStand - Get Item Property.vi"("error in (no error)"=w292, "Default Value"=FALSE, "Property Name"=w295, "Item Ref in"=w294) -> ("error out"=w291:errorcluster, "Value"=w290:bool, "Item Ref out"=w293:T5)  [unwired: 4 in, 1 out]
      n163 = case shown="False" w290 {
        tunnel: w289 -> [w345 _]
        tunnel: [w335 w357] -> w280
        tunnel: [w337 w358] -> w281
        tunnel: w293 -> [w341 w357]
        tunnel: w291 -> [w340 w358]
        tunnel: [w339 _] -> w282
        frame False {
          n164 = call <vilib>:"NI VeriStand - Get Item Parent.vi"("error in (no error)"=w340, "Item Ref in"=w341) -> ("error out"=w346:errorcluster, "Parent Ref"=w347:T5, "Item Ref out"=w342:T5)  [unwired: 6 in, 1 out]
          n165 = global read "Constants.vi" "Chassis IP Address"() -> (w330:string)
          n166 = call "SLSC Get IP Address from Chassis_O2.vi"("error in (no error)"=w346, "IP Address Global Name"=w330, "Node Ptr"=w347) -> ("error out"=w348:errorcluster, "Name or IP Address"=w349:string, "Password"=w332:string, "Username"=w333:string)  [unwired: 3 in, 2 out]
          n167 = call "SLSC Get EDS Module Information_O2.vi"("Password"=w332, "Username"=w333, "error in (no error)"=w348, "Slot #"=w345, "Chassis IP Address"=w349) -> ("error out"=w344:errorcluster, "SLSC Module Name"=w339:string, "Initialized?"=w334:bool, "SLSC EDS module"=w331:T7)  [unwired: 3 in]
          n168 = global read "Constants.vi" "initialized?"() -> (w343:string)
          n169 = call-poly <vilib>:"NI VeriStand - Set Item Property.vi"("error in (no error)"=w344, "Value"=w334, "Property Name"=w343, "Item Ref in"=w342) -> ("error out"=w338:errorcluster, "Item Ref out"=w336:T5)  [unwired: 5 in, 1 out]
          n170 = case shown="True" w334 {
            tunnel: w338 -> [w351 w356]
            tunnel: [w351 w355] -> w337
            tunnel: w336 -> [w350 w354]
            tunnel: [w350 w353] -> w335
            tunnel: w331 -> [_ w352]
            frame False {
            }
            frame True {
              n171 = call "Initialization_channels.vi"("error in (no error)"=w356, "SLSC EDS module"=w352, "Device Item Ref in"=w354) -> ("error out"=w355:errorcluster, "Device Item Ref out"=w353:T5)  [unwired: 7 in]
            }
          }
        }
        frame True {
        }
      }
      n172 = case shown="True" w290 {
        tunnel: w282 -> [w361 _]
        tunnel: [w361 w366] -> w279
        tunnel: w281 -> [w360 w370]
        tunnel: w280 -> [w359 w369]
        tunnel: [w360 w371] -> w277
        tunnel: w289 -> [_ w368]
        tunnel: [w359 w367] -> w278
        frame False {
        }
        frame True {
          n173 = call <vilib>:"NI VeriStand - Get Item Parent.vi"("error in (no error)"=w370, "Item Ref in"=w369) -> ("error out"=w372:errorcluster, "Parent Ref"=w373:T5, "Item Ref out"=w367:T5)  [unwired: 6 in, 1 out]
          n174 = global read "Constants.vi" "Chassis IP Address"() -> (w365:string)
          n175 = call "SLSC Get IP Address from Chassis_O2.vi"("error in (no error)"=w372, "IP Address Global Name"=w365, "Node Ptr"=w373) -> ("error out"=w363:errorcluster, "Name or IP Address"=w364:string)  [unwired: 3 in, 4 out]
          n176 = call "SLSC Get Module Name from IP Address_O2.vi"("connect timeout"=5.0, "Error In"=w363, "Slot #"=w368, "Chassis IP Address"=w364) -> ("Error Out"=w371:errorcluster, "SLSC Module Name"=w366:string)  [unwired: 5 in, 1 out]
        }
      }
      "SLSC Module Name" <- w279
      n177 = call-poly <vilib>:"NI VeriStand - Get Item Property.vi"("error in (no error)"=w277, "Property Name"="Par", "Item Ref in"=w278) -> ("error out"=w288:errorcluster, "Value"=w322:string, "Item Ref out"=w287:T5)  [unwired: 5 in, 1 out]
      n178 = Unflatten From String(type="par 3", binary string=w322) -> (value=w306:T2)  [unwired: 3 in, 2 out]
      n179 = Unbundle By Name(w306) -> ("Mode"=w309:enum16{"SLSC Mode", "ANALOG Mode"}, "Loop time.Period [ms]"=w329:i64, "Loop time.Processor"=w328:i32, "vendor.Num"=w283:u32, "product.Num"=w284:u32)
      "vendor.Num" <- w283
      "product.Num" <- w284
      n180 = Number To Decimal String(number=w284) -> (decimal integer string=w301:string)  [unwired: 1 in]
      n181 = Unbundle By Name(w306) -> ("O2Sensor1"=w314:T14, "O2Sensor2"=w315:T14, "O2Sensor3"=w316:T14, "O2Sensor4"=w317:T14)
      n182 = Concatenate Strings("ALMA-" ("Property Name"), w301) -> (→"Board":string)
      n183 = local read "RefArray"() -> (w319:refnum<vi>[])
      n184 = Build Array(w314, w315, w316, w317) -> (w318:T15)
      n185 = local write "Period [ms]"(w329) -> ()
      n186 = local write "Mode"(w309) -> ()
      n187 = local write "Processor"(w328) -> ()
      n188 = for {
        tunnel: w318 -> [w433] mode=indexing
        tunnel: w319 -> [w415]
        tunnel: w313 -> [w414] mode=indexing
        tunnel: w312 -> [w426] mode=indexing
        tunnel: w311 -> [w422] mode=indexing
        tunnel: w310 -> [w418] mode=indexing
        n189 = Array Subset(array=w415, index=w414, length=10 ("index")) -> (w423:refnum<vi>[])
        n190 = Array Subset(array=w415, index=w418, length=4) -> (w417:refnum<vi>[])
        n191 = Array Subset(array=w415, index=w422, length=4) -> (w420:refnum<vi>[])
        n192 = Index Array(array=w415, index=w426) -> (element=w427:refnum<vi>)
        n193 = Build Array (concatenate)(w423, w417) -> (w416:refnum<vi>[])
        n194 = Unbundle By Name(w433) -> ("Lambda Type"=w424:T3, "Lambda.LSU4.2 Lambda"=w437:dbl[], "Lambda.LSU4.2 Ip"=w438:dbl[], "Lambda.LSU4.9 Lambda"=w439:dbl[], "Lambda.LSU4.9 Ip"=w440:dbl[], "Lambda.LZA03 Lambda"=w445:dbl[], "Lambda.LZA03 Ip"=w446:dbl[], "Lambda.LZA08 Lambda"=w441:dbl[], "Lambda.LZA08 Ip"=w442:dbl[], "Lambda.Custom Lambda"=w447:dbl[], "Lambda.Custom Ip"=w448:dbl[], "Temp.LSU4.2 Temp"=w454:dbl[], "Temp.LSU4.2 Ohm"=w455:dbl[], "Temp.LSU4.9 Temp"=w456:dbl[], "Temp.LSU4.9 Ohm"=w457:dbl[], "Temp.LZA03 Temp"=w458:dbl[], "Temp.LZA03 Ohm"=w459:dbl[], "Temp.LZA08 Temp"=w460:dbl[], "Temp.LZA08 Ohm"=w461:dbl[], "Temp.Custom Temp"=w462:dbl[], "Temp.Custom Ohm"=w463:dbl[], "PID.Ki"=w432:dbl, "PID.Kp"=w431:dbl, "PID.Kd"=w430:dbl, "PID.FeedFW"=w429:dbl)
        n195 = case shown="5" w424 {
          tunnel: w416 -> [w465 w468 w472 w476 w480 w484]
          frame 0, Default {
            n196 = for {
              tunnel: w465 -> [w467] mode=indexing
              tunnel: bool[] [TRUE, FALSE, FALSE, FALSE, FALSE, TRUE, FALSE, FALSE, FALSE, FALSE, TRUE, TRUE, TRUE, TRUE] -> [w466] mode=indexing
              n197 = property class="Ctl"(reference=w467, "Visible"=w466) -> ()  [unwired: 1 in, 2 out]
            }
          }
          frame 1 {
            n198 = for {
              tunnel: w468 -> [w471] mode=indexing
              tunnel: bool[] [FALSE, TRUE, FALSE, FALSE, FALSE, FALSE, TRUE, FALSE, FALSE, FALSE, TRUE, TRUE, TRUE, TRUE] -> [w470] mode=indexing
              n199 = property class="Ctl"(reference=w471, "Visible"=w470) -> ()  [unwired: 1 in, 2 out]
            }
          }
          frame 2 {
            n200 = for {
              tunnel: w472 -> [w475] mode=indexing
              tunnel: bool[] [FALSE, FALSE, FALSE, TRUE, FALSE, FALSE, FALSE, FALSE, TRUE, FALSE, TRUE, TRUE, TRUE, TRUE] -> [w474] mode=indexing
              n201 = property class="Ctl"(reference=w475, "Visible"=w474) -> ()  [unwired: 1 in, 2 out]
            }
          }
          frame 3 {
            n202 = for {
              tunnel: w476 -> [w479] mode=indexing
              tunnel: bool[] [FALSE, FALSE, TRUE, FALSE, FALSE, FALSE, FALSE, TRUE, FALSE, FALSE, TRUE, TRUE, TRUE, TRUE] -> [w478] mode=indexing
              n203 = property class="Ctl"(reference=w479, "Visible"=w478) -> ()  [unwired: 1 in, 2 out]
            }
          }
          frame 4 {
            n204 = for {
              tunnel: w480 -> [w483] mode=indexing
              tunnel: bool[] [FALSE, FALSE, FALSE, FALSE, TRUE, FALSE, FALSE, FALSE, FALSE, TRUE, TRUE, TRUE, TRUE, TRUE] -> [w482] mode=indexing
              n205 = property class="Ctl"(reference=w483, "Visible"=w482) -> ()  [unwired: 1 in, 2 out]
            }
          }
          frame 5 {
            n206 = for {
              tunnel: w484 -> [w487] mode=indexing
              tunnel: bool[] [FALSE, FALSE, FALSE, FALSE, FALSE, FALSE, FALSE, FALSE, FALSE, FALSE, FALSE, FALSE, FALSE, FALSE] -> [w486] mode=indexing
              n207 = property class="Ctl"(reference=w487, "Visible"=w486) -> ()  [unwired: 1 in, 2 out]
            }
          }
        }
        n208 = Build Array(w432, w431, w430, w429) -> (w428:dbl[])
        n209 = for {
          tunnel: w428 -> [w489] mode=indexing
          tunnel: w420 -> [w488] mode=indexing
          n210 = property class="Ctl"(reference=w488, "Val(Sgnl)"=w489) -> ()  [unwired: 1 in, 2 out]
        }
        n211 = property class="Ctl"(reference=w427, "Val(Sgnl)"=w424) -> ()  [unwired: 1 in, 2 out]
        n212 = Build Array(w437, w438) -> (w434:dbl[][])
        n213 = Build Array(w439, w440) -> (w435:dbl[][])
        n214 = Build Array(w445, w446) -> (w444:dbl[][])
        n215 = Build Array(w441, w442) -> (w436:dbl[][])
        n216 = Index Array(array=w415, index #1=w414) -> (element #1=w413:refnum<vi>, element #2=w411:refnum<vi>, element #3=w410:refnum<vi>, element #4=w409:refnum<vi>, element #5=w408:refnum<vi>, element #6=w407:refnum<vi>, element #7=w406:refnum<vi>, element #8=w405:refnum<vi>, element #9=w404:refnum<vi>, element #10=w403:refnum<vi>)  [unwired: 9 in]
        n217 = Build Array(w447, w448) -> (w443:dbl[][])
        n218 = Build Array(w454, w455) -> (w453:dbl[][])
        n219 = Build Array(w456, w457) -> (w452:dbl[][])
        n220 = Build Array(w458, w459) -> (w449:dbl[][])
        n221 = Build Array(w460, w461) -> (w451:dbl[][])
        n222 = Build Array(w462, w463) -> (w450:dbl[][])
        n223 = Transpose 2D Array(2D array=w434) -> (transposed array=w412:dbl[][])
        n224 = Transpose 2D Array(2D array=w435) -> (transposed array=w402:dbl[][])
        n225 = Transpose 2D Array(2D array=w444) -> (transposed array=w401:dbl[][])
        n226 = Transpose 2D Array(2D array=w436) -> (transposed array=w400:dbl[][])
        n227 = Transpose 2D Array(2D array=w443) -> (transposed array=w399:dbl[][])
        n228 = Transpose 2D Array(2D array=w453) -> (transposed array=w398:dbl[][])
        n229 = Transpose 2D Array(2D array=w452) -> (transposed array=w397:dbl[][])
        n230 = Transpose 2D Array(2D array=w449) -> (transposed array=w396:dbl[][])
        n231 = Transpose 2D Array(2D array=w451) -> (transposed array=w395:dbl[][])
        n232 = Transpose 2D Array(2D array=w450) -> (transposed array=w394:dbl[][])
        n233 = property class="Ctl"(reference=w405, "Val(Sgnl)"=w396) -> ()  [unwired: 1 in, 2 out]
        n234 = property class="Ctl"(reference=w407, "Val(Sgnl)"=w398) -> ()  [unwired: 1 in, 2 out]
        n235 = property class="Ctl"(reference=w403, "Val(Sgnl)"=w394) -> ()  [unwired: 1 in, 2 out]
        n236 = property class="Ctl"(reference=w409, "Val(Sgnl)"=w400) -> ()  [unwired: 1 in, 2 out]
        n237 = property class="Ctl"(reference=w406, "Val(Sgnl)"=w397) -> ()  [unwired: 1 in, 2 out]
        n238 = property class="Ctl"(reference=w411, "Val(Sgnl)"=w402) -> ()  [unwired: 1 in, 2 out]
        n239 = property class="Ctl"(reference=w408, "Val(Sgnl)"=w399) -> ()  [unwired: 1 in, 2 out]
        n240 = property class="Ctl"(reference=w404, "Val(Sgnl)"=w395) -> ()  [unwired: 1 in, 2 out]
        n241 = property class="Ctl"(reference=w410, "Val(Sgnl)"=w401) -> ()  [unwired: 1 in, 2 out]
        n242 = property class="Ctl"(reference=w413, "Val(Sgnl)"=w412) -> ()  [unwired: 1 in, 2 out]
      }
      n243 = case shown="10201" w284 {
        frame 10201 {
          n244 = property on="Tab Control 2" class="TabCtl (strict)"() -> ("Pages"=w387:refnum<vi>[])  [unwired: 2 in, 2 out]
          n245 = for {
            tunnel: w387 -> [w389] mode=indexing
            tunnel: bool[] [TRUE, TRUE, FALSE, FALSE] -> [w388] mode=indexing
            n246 = property class="Page"(reference=w389, "PageVis"=w388) -> ()  [unwired: 1 in, 2 out]
          }
        }
        frame 10401, Default {
          n247 = property on="Tab Control 2" class="TabCtl (strict)"() -> ("Pages"=w391:refnum<vi>[])  [unwired: 2 in, 2 out]
          n248 = for {
            tunnel: w391 -> [w393] mode=indexing
            tunnel: bool[] [TRUE, TRUE, TRUE, TRUE] -> [w392] mode=indexing
            n249 = property class="Page"(reference=w393, "PageVis"=w392) -> ()  [unwired: 1 in, 2 out]
          }
        }
      }
      n250 = disable-structure shown="Enabled" {
        disable-tunnel: [w379 w385] -> w308
        disable-tunnel: [w378 w384] -> w307
        disable-tunnel: w288 -> [w377 w384]
        disable-tunnel: w287 -> [w376 w385]
        disable-tunnel: w284 -> [w375 _]
        disable-tunnel: w283 -> [w374 _]
        frame Disabled {
          n251 = global read "Constants.vi" "productNumber"() -> (w381:string)
          n252 = global read "Constants.vi" "vendorNumber"() -> (w380:string)
          n253 = call-poly <vilib>:"NI VeriStand - Set Item Property.vi"("error in (no error)"=w377, "Value"=w375, "Property Name"=w381, "Item Ref in"=w376) -> ("error out"=w383:errorcluster, "Item Ref out"=w382:T5)  [unwired: 5 in, 1 out]
          n254 = call-poly <vilib>:"NI VeriStand - Set Item Property.vi"("error in (no error)"=w383, "Value"=w374, "Property Name"=w380, "Item Ref in"=w382) -> ("error out"=w378:errorcluster, "Item Ref out"=w379:T5)  [unwired: 5 in, 1 out]
        }
        frame Enabled {
        }
      }
    }
  }
  n255 = call <vilib>:"NI VeriStand - Unset Busy Cursor.vi"("error in (no error)"=w2) -> ("error out"=w13:errorcluster)  [unwired: 10 out]
  n256 = case shown="No Error" w13 {
    selector: w13 -> [w493 w1264]
    tunnel: [w497 w1262] -> w9
    tunnel: w12 -> [w494 _]
    tunnel: w1 -> [w490 _]
    frame No Error {
      # "Never try to keep the FP of this VI open beyond the shutdown sequence.\nMake sure that the FP is closed at any time the shutdown sequence is received."
      n257 = call <vilib>:"NI VeriStand - Get Event Refnum.vi"("error in (no error)"=w493) -> ("error out"=w492:errorcluster, "Event Ref"=w491:refnum<user-event>)  [unwired: 9 out]
      n258 = register-events(error in=w492, w491) -> (reference out=w495:refnum<event-registration>, error out=w496:errorcluster)  [unwired: 1 in]
      n259 = while {
        tunnel: w494 -> [w537]
        shift-right: [w534] -> w498
        shift-left: w496 -> [w540]
        shift-right: [w541] -> w499
        shift-left: w495 -> [w539]
        tunnel: w490 -> [w506]
        i -> [w530]
        stop <- w538 stop-if-true
        w509 = i32[] [64, 68, 72, 76]  # PID
        w510 = i32[] [56, 57, 58, 59]  # lambda type
        w511 = i32[] [0, 10, 20, 30]  # offset
        n260 = local read "Tab Control 2"() -> (w503:T4)
        n261 = call-poly <userlib>:"Data Changed__ogtk.vi"("I32"=w503) -> ("Changed"=w502:bool)
        n262 = Equal?(x=1, y=w530) -> (x = y?=w531:bool)
        n263 = local read "RefArray"() -> (w512:refnum<vi>[])
        n264 = Unbundle By Name(w506) -> ("O2Sensor1"=w516:T14, "O2Sensor2"=w515:T14, "O2Sensor3"=w514:T14, "O2Sensor4"=w513:T14)
        n265 = Build Array(w516, w515, w514, w513) -> (w521:T15)
        n266 = for {
          tunnel: w512 -> [w608]
          tunnel: w511 -> [w670] mode=indexing
          tunnel: w521 -> [w619] mode=indexing
          tunnel: [w618] -> w505 mode=indexing
          tunnel: w510 -> [w616] mode=indexing
          tunnel: w509 -> [w607] mode=indexing
          w599 = 0.0 ("PID.Ki_1")
          w613 = T3 0 items=["LSU4.2", "LSU4.9", "LZA03", "LZA08", "Custom", "[mA]"] ("O2Sensor Type")
          w617 = dbl[][] [] ("Caratteristica LSU4.2")
          n267 = Index Array(array=w608, index #1=w607) -> (element #1=w603:refnum<vi>, element #2=w602:refnum<vi>, element #3=w601:refnum<vi>, element #4=w600:refnum<vi>)  [unwired: 3 in]
          n268 = Index Array(array=w608, index=w616) -> (element=w614:refnum<vi>)
          n269 = Index Array(array=w608, index #1=w670) -> (element #1=w665:refnum<vi>, element #2=w640:refnum<vi>, element #3=w639:refnum<vi>, element #4=w638:refnum<vi>, element #5=w637:refnum<vi>, element #6=w636:refnum<vi>, element #7=w635:refnum<vi>, element #8=w626:refnum<vi>, element #9=w625:refnum<vi>, element #10=w620:refnum<vi>)  [unwired: 9 in]
          n270 = property class="Ctl"(reference=w614) -> ("Value"=w615:variant)  [unwired: 1 in, 2 out]
          n271 = property class="Ctl"(reference=w638) -> ("Value"=w653:variant)  [unwired: 1 in, 2 out]
          n272 = property class="Ctl"(reference=w665) -> ("Value"=w669:variant)  [unwired: 1 in, 2 out]
          n273 = property class="Ctl"(reference=w600) -> ("Value"=w604:variant)  [unwired: 1 in, 2 out]
          n274 = property class="Ctl"(reference=w639) -> ("Value"=w660:variant)  [unwired: 1 in, 2 out]
          n275 = property class="Ctl"(reference=w626) -> ("Value"=w631:variant)  [unwired: 1 in, 2 out]
          n276 = property class="Ctl"(reference=w635) -> ("Value"=w644:variant)  [unwired: 1 in, 2 out]
          n277 = property class="Ctl"(reference=w602) -> ("Value"=w606:variant)  [unwired: 1 in, 2 out]
          n278 = property class="Ctl"(reference=w601) -> ("Value"=w605:variant)  [unwired: 1 in, 2 out]
          n279 = property class="Ctl"(reference=w640) -> ("Value"=w661:variant)  [unwired: 1 in, 2 out]
          n280 = property class="Ctl"(reference=w637) -> ("Value"=w652:variant)  [unwired: 1 in, 2 out]
          n281 = property class="Ctl"(reference=w603) -> ("Value"=w609:variant)  [unwired: 1 in, 2 out]
          n282 = property class="Ctl"(reference=w625) -> ("Value"=w630:variant)  [unwired: 1 in, 2 out]
          n283 = property class="Ctl"(reference=w636) -> ("Value"=w645:variant)  [unwired: 1 in, 2 out]
          n284 = property class="Ctl"(reference=w620) -> ("Value"=w621:variant)  [unwired: 1 in, 2 out]
          n285 = Variant To Data(type=w613, Variant=w615) -> (data=w612:T3)  [unwired: 1 in, 1 out]
          n286 = Variant To Data(type=w617, Variant=w653) -> (data=w656:dbl[][])  [unwired: 1 in, 1 out]
          n287 = Variant To Data(type=w617, Variant=w669) -> (data=w666:dbl[][])  [unwired: 1 in, 1 out]
          n288 = Variant To Data(type=w599, Variant=w604) -> (data=w577:dbl)  [unwired: 1 in, 1 out]
          n289 = Variant To Data(type=w617, Variant=w660) -> (data=w657:dbl[][])  [unwired: 1 in, 1 out]
          n290 = Variant To Data(type=w617, Variant=w631) -> (data=w634:dbl[][])  [unwired: 1 in, 1 out]
          n291 = Variant To Data(type=w617, Variant=w644) -> (data=w641:dbl[][])  [unwired: 1 in, 1 out]
          n292 = Variant To Data(type=w599, Variant=w606) -> (data=w579:dbl)  [unwired: 1 in, 1 out]
          n293 = Variant To Data(type=w599, Variant=w605) -> (data=w578:dbl)  [unwired: 1 in, 1 out]
          n294 = Variant To Data(type=w617, Variant=w661) -> (data=w664:dbl[][])  [unwired: 1 in, 1 out]
          n295 = Variant To Data(type=w617, Variant=w652) -> (data=w649:dbl[][])  [unwired: 1 in, 1 out]
          n296 = Variant To Data(type=w599, Variant=w609) -> (data=w580:dbl)  [unwired: 1 in, 1 out]
          n297 = Variant To Data(type=w617, Variant=w630) -> (data=w627:dbl[][])  [unwired: 1 in, 1 out]
          n298 = Variant To Data(type=w617, Variant=w645) -> (data=w648:dbl[][])  [unwired: 1 in, 1 out]
          n299 = Variant To Data(type=w617, Variant=w621) -> (data=w624:dbl[][])  [unwired: 1 in, 1 out]
          n300 = Index Array(array=w656, index (col) #1=0 ("disabled index (col)"), index (col) #2=1 ("index (col)")) -> (element #1=w594:dbl[], element #2=w593:dbl[])  [unwired: 2 in]
          n301 = Index Array(array=w666, index (col) #1=0 ("disabled index (col)"), index (col) #2=1 ("index (col)")) -> (element #1=w611:dbl[], element #2=w610:dbl[])  [unwired: 2 in]
          n302 = Index Array(array=w657, index (col) #1=0 ("disabled index (col)"), index (col) #2=1 ("index (col)")) -> (element #1=w596:dbl[], element #2=w595:dbl[])  [unwired: 2 in]
          n303 = Index Array(array=w634, index (col) #1=0 ("disabled index (col)"), index (col) #2=1 ("index (col)")) -> (element #1=w586:dbl[], element #2=w585:dbl[])  [unwired: 2 in]
          n304 = Index Array(array=w641, index (col) #1=0 ("disabled index (col)"), index (col) #2=1 ("index (col)")) -> (element #1=w588:dbl[], element #2=w587:dbl[])  [unwired: 2 in]
          n305 = Index Array(array=w664, index (col) #1=0 ("disabled index (col)"), index (col) #2=1 ("index (col)")) -> (element #1=w598:dbl[], element #2=w597:dbl[])  [unwired: 2 in]
          n306 = Index Array(array=w649, index (col) #1=0 ("disabled index (col)"), index (col) #2=1 ("index (col)")) -> (element #1=w592:dbl[], element #2=w591:dbl[])  [unwired: 2 in]
          n307 = Index Array(array=w627, index (col) #1=0 ("disabled index (col)"), index (col) #2=1 ("index (col)")) -> (element #1=w584:dbl[], element #2=w583:dbl[])  [unwired: 2 in]
          n308 = Index Array(array=w648, index (col) #1=0 ("disabled index (col)"), index (col) #2=1 ("index (col)")) -> (element #1=w590:dbl[], element #2=w589:dbl[])  [unwired: 2 in]
          n309 = Index Array(array=w624, index (col) #1=0 ("disabled index (col)"), index (col) #2=1 ("index (col)")) -> (element #1=w582:dbl[], element #2=w581:dbl[])  [unwired: 2 in]
          n310 = Bundle By Name(cluster=w619, "Lambda Type"=w612, "Lambda.LSU4.2 Lambda"=w611, "Lambda.LSU4.2 Ip"=w610, "Lambda.LSU4.9 Lambda"=w598, "Lambda.LSU4.9 Ip"=w597, "Lambda.LZA03 Lambda"=w596, "Lambda.LZA03 Ip"=w595, "Lambda.LZA08 Lambda"=w594, "Lambda.LZA08 Ip"=w593, "Lambda.Custom Lambda"=w592, "Lambda.Custom Ip"=w591, "Temp.LSU4.2 Temp"=w590, "Temp.LSU4.2 Ohm"=w589, "Temp.LSU4.9 Temp"=w588, "Temp.LSU4.9 Ohm"=w587, "Temp.LZA03 Temp"=w586, "Temp.LZA03 Ohm"=w585, "Temp.LZA08 Temp"=w584, "Temp.LZA08 Ohm"=w583, "Temp.Custom Temp"=w582, "Temp.Custom Ohm"=w581, "PID.Ki"=w580, "PID.Kp"=w579, "PID.Kd"=w578, "PID.FeedFW"=w577) -> (w618:T14)
        }
        n311 = Index Array(array=w505) -> (element #1=w520:T14, element #2=w519:T14, element #3=w518:T14, element #4=w517:T14)  [unwired: 4 in]
        n312 = In Range and Coerce(upper limit=i64 100, x="Period [ms]", lower limit=i64 1) -> (coerced(x)=w524:i64)  [unwired: 1 out]
        n313 = Bundle By Name(cluster=w506, "O2Sensor1"=w520, "O2Sensor2"=w519, "O2Sensor3"=w518, "O2Sensor4"=w517) -> (w508:T2)
        n314 = local write "Period [ms]"(w524) -> ()
        n315 = Bundle By Name(cluster=w508, "Mode"="Mode", "Loop time.Period [ms]"=w524, "Loop time.Processor"="Processor", "COM.COM port"=u64 30005 ("Local port"), "COM.Local port"=u64 5556 ("Lambda port")) -> (w527:T2)
        n316 = event shown="[1] \"Name\": Value Change" {
          selector: w539 -> [_ _ _ _ _ _ _ _ _ _]
          dyn-events: [_ _ _ _ _ _ _ _ _ _] -> w541
          timeout: 100 -> [_ _ _ _ _ _ _ _ _ _]
          tunnel: w540 -> [w679 w709 w712 w714 w727 w763 w886 w1009 w1132 w1255]
          tunnel: [w675 _ _ _ _ _ _ _ _ _] -> w538
          tunnel: [w674 w708 w711 w714 w728 w770 w893 w1016 w1139 w1254] -> w536
          tunnel: w537 -> [w673 w707 w713 _ w726 w769 w892 w1015 w1138 _]
          tunnel: w527 -> [_ _ _ _ w715 w768 w891 w1014 w1137 _]
          event User Event {
            n317 = event-data() -> ("Data"=w678:string)  [unwired: 1 out]
            n318 = call <vilib>:"NI VeriStand - Parse Incoming Command Data.vi"("error in (no error)"=w679, "Incoming data"=w678) -> ("error out"=w677:errorcluster, "Outgoing data"=w672:variant, "Action"=w676:T17)  [unwired: 7 out]
            n319 = case shown="\"Dynamic button pressed\"" w676 {
              tunnel: w677 -> [w680 w685 w686 w693]
              tunnel: [_ _ TRUE _] -> w675
              tunnel: [w680 w682 w686 w688] -> w674
              tunnel: w673 -> [_ w684 _ _]
              tunnel: w672 -> [_ _ _ w692]
              frame "Default", Default {
              }
              frame "Item renamed" {
                n320 = call <vilib>:"NI VeriStand - Get Item Data.vi"("error in (no error)"=w685, "Item Ref in"=w684) -> ("error out"=w682:errorcluster, "Item Info"=w683:T6)  [unwired: 8 out]
                n321 = Unbundle By Name(w683) -> ("Name"=w681:string)
                n322 = local write "Name"(w681) -> ()
              }
              frame "Shutdown" {
                # "The page has received the command to save all its data and to acknowledge that the page is ready to get unloaded from memory."
              }
              frame "Dynamic button pressed" {
                w691 = ""  # Button ID
                n323 = Variant To Data(error in=w693, type=w691, Variant=w692) -> (data=w690:string, error out=w689:errorcluster)
                n324 = case shown="\"Diagram\", \"Pinout\"" w690 {
                  selector: w690 -> [_ w703]
                  tunnel: w689 -> [w694 w705]
                  tunnel: [w694 w704] -> w688
                  frame Default {
                  }
                  frame "Diagram", "Pinout" {
                    # "Open and forget..."
                    n325 = vi-ref "Read_image.vi"() -> (w696:refnum<vi>)
                    n326 = property class="VI Interface Type 0"(reference=w696) -> ("Name"=w697:string)  [unwired: 1 in, 2 out]
                    n327 = local read "product.Num"() -> (w695:u32)
                    n328 = Open VI Reference(type specifier VI Refnum (for type only)=w696, vi path=w697, options=128, error in (no error)=w705) -> (vi reference=w701:refnum<vi>, error out=w699:errorcluster)  [unwired: 2 in]
                    n329 = call-by-ref "Start Asynchronous Call"(reference=w701, error in=w699, "Type"=w703, "ProductNum"=w695) -> (reference out=w700:refnum<vi>, error out=w698:errorcluster)  [unwired: 10 in]
                    n330 = Close Reference(reference=w700, error in (no error)=w698) -> (error out=w704:errorcluster)
                  }
                }
              }
            }
          }
          event "Name": Value Change {
            n331 = event-data() -> ()  [unwired: 2 out]
            n332 = call <vilib>:"NI VeriStand - Rename Custom Device Item.vi"("error in (no error)"=w709, "New Name"="Name", "Item Ref in"=w707) -> ("error out"=w708:errorcluster)  [unwired: 1 in, 7 out]
          }
          event "Description": Value Change {
            n333 = event-data() -> ()  [unwired: 2 out]
            n334 = call <vilib>:"NI VeriStand - Set Item Description.vi"("error in (no error)"=w712, "Description"="Description", "Item Ref in"=w713) -> ("error out"=w711:errorcluster)  [unwired: 8 out]
          }
          event Timeout {
            n335 = event-data() -> ()  [unwired: 4 out]
          }
          event "ParamUpdate": Value Change {
            w722 = i32[] [40, 44, 48, 52]  # lable
            w721 = i32[] [0, 10, 20, 30]  # offset
            n336 = event-data() -> ()  [unwired: 2 out]
            n337 = Unbundle By Name(w715) -> ("O2Sensor1.Lambda Type"=w716:T3, "O2Sensor2.Lambda Type"=w717:T3, "O2Sensor3.Lambda Type"=w718:T3, "O2Sensor4.Lambda Type"=w719:T3)
            n338 = Build Array(w716, w717, w718, w719) -> (w720:T3[])
            n339 = for {
              tunnel: w720 -> [w731] mode=indexing
              tunnel: w721 -> [w730] mode=indexing
              tunnel: w722 -> [w729] mode=indexing
              n340 = local read "RefArray"() -> (w735:refnum<vi>[])
              n341 = Array Subset(array=w735, index=w729, length=4) -> (w736:refnum<vi>[])
              n342 = Array Subset(array=w735, index=w730, length=10 ("index")) -> (w737:refnum<vi>[])
              n343 = Build Array (concatenate)(w737, w736) -> (w734:refnum<vi>[])
              n344 = case shown="0, Default" w731 {
                tunnel: w734 -> [w739 w742 w746 w750 w754 w758]
                frame 0, Default {
                  n345 = for {
                    tunnel: w739 -> [w741] mode=indexing
                    tunnel: bool[] [TRUE, FALSE, FALSE, FALSE, FALSE, TRUE, FALSE, FALSE, FALSE, FALSE, TRUE, TRUE, TRUE, TRUE] -> [w740] mode=indexing
                    n346 = property class="Ctl"(reference=w741, "Visible"=w740) -> ()  [unwired: 1 in, 2 out]
                  }
                }
                frame 1 {
                  n347 = for {
                    tunnel: w742 -> [w745] mode=indexing
                    tunnel: bool[] [FALSE, TRUE, FALSE, FALSE, FALSE, FALSE, TRUE, FALSE, FALSE, FALSE, TRUE, TRUE, TRUE, TRUE] -> [w744] mode=indexing
                    n348 = property class="Ctl"(reference=w745, "Visible"=w744) -> ()  [unwired: 1 in, 2 out]
                  }
                }
                frame 2 {
                  n349 = for {
                    tunnel: w746 -> [w749] mode=indexing
                    tunnel: bool[] [FALSE, FALSE, FALSE, TRUE, FALSE, FALSE, FALSE, FALSE, TRUE, FALSE, TRUE, TRUE, TRUE, TRUE] -> [w748] mode=indexing
                    n350 = property class="Ctl"(reference=w749, "Visible"=w748) -> ()  [unwired: 1 in, 2 out]
                  }
                }
                frame 3 {
                  n351 = for {
                    tunnel: w750 -> [w753] mode=indexing
                    tunnel: bool[] [FALSE, FALSE, TRUE, FALSE, FALSE, FALSE, FALSE, TRUE, FALSE, FALSE, TRUE, TRUE, TRUE, TRUE] -> [w752] mode=indexing
                    n352 = property class="Ctl"(reference=w753, "Visible"=w752) -> ()  [unwired: 1 in, 2 out]
                  }
                }
                frame 4 {
                  n353 = for {
                    tunnel: w754 -> [w757] mode=indexing
                    tunnel: bool[] [FALSE, FALSE, FALSE, FALSE, TRUE, FALSE, FALSE, FALSE, FALSE, TRUE, TRUE, TRUE, TRUE, TRUE] -> [w756] mode=indexing
                    n354 = property class="Ctl"(reference=w757, "Visible"=w756) -> ()  [unwired: 1 in, 2 out]
                  }
                }
                frame 5 {
                  n355 = for {
                    tunnel: w758 -> [w761] mode=indexing
                    tunnel: bool[] [FALSE, FALSE, FALSE, FALSE, FALSE, FALSE, FALSE, FALSE, FALSE, FALSE, FALSE, FALSE, FALSE, FALSE] -> [w760] mode=indexing
                    n356 = property class="Ctl"(reference=w761, "Visible"=w760) -> ()  [unwired: 1 in, 2 out]
                  }
                }
              }
            }
            n357 = Flatten To String(anything=w715, error in (no error)=w727) -> (data string=w723:string, error out=w724:errorcluster)  [unwired: 2 in, 1 out]
            n358 = call-poly <vilib>:"NI VeriStand - Set Item Property.vi"("error in (no error)"=w724, "Value"=w723, "Property Name"="Par", "Item Ref in"=w726) -> ("error out"=w728:errorcluster)  [unwired: 5 in, 2 out]
          }
          event "Import": Value Change {
            n359 = event-data() -> ()  [unwired: 7 out]
            n360 = Unbundle By Name(w768) -> ("O2Sensor1.Lambda Type"=w767:T3)
            n361 = Open/Create/Replace File(error in=w763, operation (0:open)=T16."open", access (0:read/write)=enum16{"read/write", "read-only", "write-only"}."read-only") -> (refnum out=w766:refnum<file>, error out=w762:errorcluster)  [unwired: 3 in, 1 out]
            n362 = case shown="No Error" w762 {
              selector: w762 -> [w784 w884]
              tunnel: [w808 w883] -> w770
              tunnel: w769 -> [w807 _]
              tunnel: w768 -> [w803 _]
              tunnel: w767 -> [w773 _]
              tunnel: w766 -> [w800 _]
              frame No Error {
                w782 = 0 ("index")
                n363 = Read from Text File(file (use dialog)=w800, error in=w784) -> (refnum out=w801:refnum<file>, text=w799:string, error out=w802:errorcluster)  [unwired: 2 in, 1 out]
                n364 = Spreadsheet String To Array(delimiter (Tab)=",", format string="%s", spreadsheet string=w799) -> (array=w791:dbl[][])  [unwired: 1 in]
                n365 = Close File(refnum=w801, error in=w802) -> ()  [unwired: 2 out]
                n366 = Delete From Array(array=w791, length=1, index (row)=0) -> (array with subset deleted=w793:dbl[][])  [unwired: 1 in, 1 out]
                n367 = Index Array(array=w793, index (col) #1=0 ("disabled index (col)"), index (col) #2=1 ("index (col)")) -> (element #1=w794:dbl[], element #2=w795:dbl[], element #3=w788:dbl[], element #4=w789:dbl[])  [unwired: 6 in]
                n368 = Build Array(w789, w788) -> (w790:dbl[][])
                n369 = Build Array(w795, w794) -> (w796:dbl[][])
                n370 = Transpose 2D Array(2D array=w790) -> (transposed array=w771:dbl[][])
                n371 = Transpose 2D Array(2D array=w796) -> (transposed array=w772:dbl[][])
                n372 = local read "RefArray"() -> (w780:refnum<vi>[])
                n373 = Add(x=w782, y=5) -> (x+y=w781:i32)
                n374 = Array Subset(array=w780, index=40, length=4) -> (w775:refnum<vi>[])
                n375 = Array Subset(array=w780, index=w782, length=10 ("index")) -> (w774:refnum<vi>[])
                n376 = Build Array (concatenate)(w774, w775) -> (w776:refnum<vi>[])
                n377 = case shown="0, Default" w773 {
                  tunnel: w776 -> [w820 w833 w847 w861 w875 w879]
                  tunnel: w780 -> [w818 w827 w841 w855 w869 _]
                  tunnel: w782 -> [w815 w826 w840 w854 w868 _]
                  tunnel: w781 -> [w813 w825 w839 w853 w867 _]
                  tunnel: w772 -> [w810 w824 w838 w852 w866 _]
                  tunnel: w771 -> [w809 w823 w837 w851 w865 _]
                  frame 0, Default {
                    w814 = 0 ("y")
                    n378 = Add(x=w813, y=w814) -> (x+y=w811:i32)
                    n379 = Add(x=w815, y=w814) -> (x+y=w812:i32)
                    n380 = for {
                      tunnel: w820 -> [w822] mode=indexing
                      tunnel: bool[] [TRUE, FALSE, FALSE, FALSE, FALSE, TRUE, FALSE, FALSE, FALSE, FALSE, TRUE, TRUE, TRUE, TRUE] -> [w821] mode=indexing
                      n381 = property class="Ctl"(reference=w822, "Visible"=w821) -> ()  [unwired: 1 in, 2 out]
                    }
                    n382 = Index Array(array=w818, index #1=w812, index #2=w811) -> (element #1=w817:refnum<vi>, element #2=w816:refnum<vi>)
                    n383 = property class="Ctl"(reference=w816, "Val(Sgnl)"=w809) -> ()  [unwired: 1 in, 2 out]
                    n384 = property class="Ctl"(reference=w817, "Val(Sgnl)"=w810) -> ()  [unwired: 1 in, 2 out]
                  }
                  frame 1 {
                    w830 = 1 ("y")
                    n385 = Add(x=w825, y=w830) -> (x+y=w828:i32)
                    n386 = Add(x=w826, y=w830) -> (x+y=w829:i32)
                    n387 = Index Array(array=w827, index #1=w829, index #2=w828) -> (element #1=w832:refnum<vi>, element #2=w831:refnum<vi>)
                    n388 = for {
                      tunnel: w833 -> [w836] mode=indexing
                      tunnel: bool[] [FALSE, TRUE, FALSE, FALSE, FALSE, FALSE, TRUE, FALSE, FALSE, FALSE, TRUE, TRUE, TRUE, TRUE] -> [w835] mode=indexing
                      n389 = property class="Ctl"(reference=w836, "Visible"=w835) -> ()  [unwired: 1 in, 2 out]
                    }
                    n390 = property class="Ctl"(reference=w831, "Val(Sgnl)"=w823) -> ()  [unwired: 1 in, 2 out]
                    n391 = property class="Ctl"(reference=w832, "Val(Sgnl)"=w824) -> ()  [unwired: 1 in, 2 out]
                  }
                  frame 2 {
                    w844 = 2 ("y")
                    n392 = Add(x=w839, y=w844) -> (x+y=w842:i32)
                    n393 = Add(x=w840, y=w844) -> (x+y=w843:i32)
                    n394 = Index Array(array=w841, index #1=w843, index #2=w842) -> (element #1=w846:refnum<vi>, element #2=w845:refnum<vi>)
                    n395 = for {
                      tunnel: w847 -> [w850] mode=indexing
                      tunnel: bool[] [FALSE, FALSE, FALSE, TRUE, FALSE, FALSE, FALSE, FALSE, TRUE, FALSE, TRUE, TRUE, TRUE, TRUE] -> [w849] mode=indexing
                      n396 = property class="Ctl"(reference=w850, "Visible"=w849) -> ()  [unwired: 1 in, 2 out]
                    }
                    n397 = property class="Ctl"(reference=w845, "Val(Sgnl)"=w837) -> ()  [unwired: 1 in, 2 out]
                    n398 = property class="Ctl"(reference=w846, "Val(Sgnl)"=w838) -> ()  [unwired: 1 in, 2 out]
                  }
                  frame 3 {
                    w858 = 3 ("y")
                    n399 = Add(x=w853, y=w858) -> (x+y=w856:i32)
                    n400 = Add(x=w854, y=w858) -> (x+y=w857:i32)
                    n401 = Index Array(array=w855, index #1=w857, index #2=w856) -> (element #1=w860:refnum<vi>, element #2=w859:refnum<vi>)
                    n402 = for {
                      tunnel: w861 -> [w864] mode=indexing
                      tunnel: bool[] [FALSE, FALSE, TRUE, FALSE, FALSE, FALSE, FALSE, TRUE, FALSE, FALSE, TRUE, TRUE, TRUE, TRUE] -> [w863] mode=indexing
                      n403 = property class="Ctl"(reference=w864, "Visible"=w863) -> ()  [unwired: 1 in, 2 out]
                    }
                    n404 = property class="Ctl"(reference=w859, "Val(Sgnl)"=w851) -> ()  [unwired: 1 in, 2 out]
                    n405 = property class="Ctl"(reference=w860, "Val(Sgnl)"=w852) -> ()  [unwired: 1 in, 2 out]
                  }
                  frame 4 {
                    w870 = 4 ("y")
                    n406 = Add(x=w867, y=w870) -> (x+y=w871:i32)
                    n407 = Add(x=w868, y=w870) -> (x+y=w872:i32)
                    n408 = Index Array(array=w869, index #1=w872, index #2=w871) -> (element #1=w874:refnum<vi>, element #2=w873:refnum<vi>)
                    n409 = for {
                      tunnel: w875 -> [w878] mode=indexing
                      tunnel: bool[] [FALSE, FALSE, FALSE, FALSE, TRUE, FALSE, FALSE, FALSE, FALSE, TRUE, TRUE, TRUE, TRUE, TRUE] -> [w877] mode=indexing
                      n410 = property class="Ctl"(reference=w878, "Visible"=w877) -> ()  [unwired: 1 in, 2 out]
                    }
                    n411 = property class="Ctl"(reference=w873, "Val(Sgnl)"=w865) -> ()  [unwired: 1 in, 2 out]
                    n412 = property class="Ctl"(reference=w874, "Val(Sgnl)"=w866) -> ()  [unwired: 1 in, 2 out]
                  }
                  frame 5 {
                    n413 = for {
                      tunnel: w879 -> [w882] mode=indexing
                      tunnel: bool[] [FALSE, FALSE, FALSE, FALSE, FALSE, FALSE, FALSE, FALSE, FALSE, FALSE, FALSE, FALSE, FALSE, FALSE] -> [w881] mode=indexing
                      n414 = property class="Ctl"(reference=w882, "Visible"=w881) -> ()  [unwired: 1 in, 2 out]
                    }
                  }
                }
                n415 = Flatten To String(anything=w803) -> (data string=w804:string, error out=w805:errorcluster)  [unwired: 3 in, 1 out]
                n416 = call-poly <vilib>:"NI VeriStand - Set Item Property.vi"("error in (no error)"=w805, "Value"=w804, "Property Name"="Par", "Item Ref in"=w807) -> ("error out"=w808:errorcluster)  [unwired: 5 in, 2 out]
              }
              frame Error {
                n417 = call <vilib>:"Clear Errors.vi"("error in (no error)"=w884) -> ("error out"=w883:errorcluster)  [unwired: 5 in, 1 out]
              }
            }
          }
          event "Import 2": Value Change {
            n418 = event-data() -> ()  [unwired: 7 out]
            n419 = Unbundle By Name(w891) -> ("O2Sensor2.Lambda Type"=w890:T3)
            n420 = Open/Create/Replace File(error in=w886, operation (0:open)=T16."open", access (0:read/write)=enum16{"read/write", "read-only", "write-only"}."read-only") -> (refnum out=w889:refnum<file>, error out=w885:errorcluster)  [unwired: 3 in, 1 out]
            n421 = case shown="No Error" w885 {
              selector: w885 -> [w907 w1007]
              tunnel: [w931 w1006] -> w893
              tunnel: w892 -> [w930 _]
              tunnel: w891 -> [w926 _]
              tunnel: w890 -> [w896 _]
              tunnel: w889 -> [w923 _]
              frame No Error {
                w905 = 10 ("index")
                n422 = Read from Text File(file (use dialog)=w923, error in=w907) -> (refnum out=w924:refnum<file>, text=w922:string, error out=w925:errorcluster)  [unwired: 2 in, 1 out]
                n423 = Spreadsheet String To Array(delimiter (Tab)=",", format string="%s", spreadsheet string=w922) -> (array=w914:dbl[][])  [unwired: 1 in]
                n424 = Close File(refnum=w924, error in=w925) -> ()  [unwired: 2 out]
                n425 = Delete From Array(array=w914, length=1, index (row)=0) -> (array with subset deleted=w916:dbl[][])  [unwired: 1 in, 1 out]
                n426 = Index Array(array=w916, index (col) #1=0 ("disabled index (col)"), index (col) #2=1 ("index (col)")) -> (element #1=w917:dbl[], element #2=w918:dbl[], element #3=w911:dbl[], element #4=w912:dbl[])  [unwired: 6 in]
                n427 = Build Array(w912, w911) -> (w913:dbl[][])
                n428 = Build Array(w918, w917) -> (w919:dbl[][])
                n429 = Transpose 2D Array(2D array=w913) -> (transposed array=w894:dbl[][])
                n430 = Transpose 2D Array(2D array=w919) -> (transposed array=w895:dbl[][])
                n431 = local read "RefArray"() -> (w903:refnum<vi>[])
                n432 = Add(x=w905, y=5) -> (x+y=w904:i32)
                n433 = Array Subset(array=w903, index=44, length=4) -> (w898:refnum<vi>[])
                n434 = Array Subset(array=w903, index=w905, length=10 ("index")) -> (w897:refnum<vi>[])
                n435 = Build Array (concatenate)(w897, w898) -> (w899:refnum<vi>[])
                n436 = case shown="1" w896 {
                  tunnel: w899 -> [w943 w956 w970 w984 w998 w1002]
                  tunnel: w903 -> [w941 w950 w964 w978 w992 _]
                  tunnel: w905 -> [w938 w949 w963 w977 w991 _]
                  tunnel: w904 -> [w936 w948 w962 w976 w990 _]
                  tunnel: w895 -> [w933 w947 w961 w975 w989 _]
                  tunnel: w894 -> [w932 w946 w960 w974 w988 _]
                  frame 0, Default {
                    w937 = 0 ("y")
                    n437 = Add(x=w936, y=w937) -> (x+y=w934:i32)
                    n438 = Add(x=w938, y=w937) -> (x+y=w935:i32)
                    n439 = for {
                      tunnel: w943 -> [w945] mode=indexing
                      tunnel: bool[] [TRUE, FALSE, FALSE, FALSE, FALSE, TRUE, FALSE, FALSE, FALSE, FALSE, TRUE, TRUE, TRUE, TRUE] -> [w944] mode=indexing
                      n440 = property class="Ctl"(reference=w945, "Visible"=w944) -> ()  [unwired: 1 in, 2 out]
                    }
                    n441 = Index Array(array=w941, index #1=w935, index #2=w934) -> (element #1=w940:refnum<vi>, element #2=w939:refnum<vi>)
                    n442 = property class="Ctl"(reference=w939, "Val(Sgnl)"=w932) -> ()  [unwired: 1 in, 2 out]
                    n443 = property class="Ctl"(reference=w940, "Val(Sgnl)"=w933) -> ()  [unwired: 1 in, 2 out]
                  }
                  frame 1 {
                    w953 = 1 ("y")
                    n444 = Add(x=w948, y=w953) -> (x+y=w951:i32)
                    n445 = Add(x=w949, y=w953) -> (x+y=w952:i32)
                    n446 = Index Array(array=w950, index #1=w952, index #2=w951) -> (element #1=w955:refnum<vi>, element #2=w954:refnum<vi>)
                    n447 = for {
                      tunnel: w956 -> [w959] mode=indexing
                      tunnel: bool[] [FALSE, TRUE, FALSE, FALSE, FALSE, FALSE, TRUE, FALSE, FALSE, FALSE, TRUE, TRUE, TRUE, TRUE] -> [w958] mode=indexing
                      n448 = property class="Ctl"(reference=w959, "Visible"=w958) -> ()  [unwired: 1 in, 2 out]
                    }
                    n449 = property class="Ctl"(reference=w954, "Val(Sgnl)"=w946) -> ()  [unwired: 1 in, 2 out]
                    n450 = property class="Ctl"(reference=w955, "Val(Sgnl)"=w947) -> ()  [unwired: 1 in, 2 out]
                  }
                  frame 2 {
                    w967 = 2 ("y")
                    n451 = Add(x=w962, y=w967) -> (x+y=w965:i32)
                    n452 = Add(x=w963, y=w967) -> (x+y=w966:i32)
                    n453 = Index Array(array=w964, index #1=w966, index #2=w965) -> (element #1=w969:refnum<vi>, element #2=w968:refnum<vi>)
                    n454 = for {
                      tunnel: w970 -> [w973] mode=indexing
                      tunnel: bool[] [FALSE, FALSE, FALSE, TRUE, FALSE, FALSE, FALSE, FALSE, TRUE, FALSE, TRUE, TRUE, TRUE, TRUE] -> [w972] mode=indexing
                      n455 = property class="Ctl"(reference=w973, "Visible"=w972) -> ()  [unwired: 1 in, 2 out]
                    }
                    n456 = property class="Ctl"(reference=w968, "Val(Sgnl)"=w960) -> ()  [unwired: 1 in, 2 out]
                    n457 = property class="Ctl"(reference=w969, "Val(Sgnl)"=w961) -> ()  [unwired: 1 in, 2 out]
                  }
                  frame 3 {
                    w981 = 3 ("y")
                    n458 = Add(x=w976, y=w981) -> (x+y=w979:i32)
                    n459 = Add(x=w977, y=w981) -> (x+y=w980:i32)
                    n460 = Index Array(array=w978, index #1=w980, index #2=w979) -> (element #1=w983:refnum<vi>, element #2=w982:refnum<vi>)
                    n461 = for {
                      tunnel: w984 -> [w987] mode=indexing
                      tunnel: bool[] [FALSE, FALSE, TRUE, FALSE, FALSE, FALSE, FALSE, TRUE, FALSE, FALSE, TRUE, TRUE, TRUE, TRUE] -> [w986] mode=indexing
                      n462 = property class="Ctl"(reference=w987, "Visible"=w986) -> ()  [unwired: 1 in, 2 out]
                    }
                    n463 = property class="Ctl"(reference=w982, "Val(Sgnl)"=w974) -> ()  [unwired: 1 in, 2 out]
                    n464 = property class="Ctl"(reference=w983, "Val(Sgnl)"=w975) -> ()  [unwired: 1 in, 2 out]
                  }
                  frame 4 {
                    w993 = 4 ("y")
                    n465 = Add(x=w990, y=w993) -> (x+y=w994:i32)
                    n466 = Add(x=w991, y=w993) -> (x+y=w995:i32)
                    n467 = Index Array(array=w992, index #1=w995, index #2=w994) -> (element #1=w997:refnum<vi>, element #2=w996:refnum<vi>)
                    n468 = for {
                      tunnel: w998 -> [w1001] mode=indexing
                      tunnel: bool[] [FALSE, FALSE, FALSE, FALSE, TRUE, FALSE, FALSE, FALSE, FALSE, TRUE, TRUE, TRUE, TRUE, TRUE] -> [w1000] mode=indexing
                      n469 = property class="Ctl"(reference=w1001, "Visible"=w1000) -> ()  [unwired: 1 in, 2 out]
                    }
                    n470 = property class="Ctl"(reference=w996, "Val(Sgnl)"=w988) -> ()  [unwired: 1 in, 2 out]
                    n471 = property class="Ctl"(reference=w997, "Val(Sgnl)"=w989) -> ()  [unwired: 1 in, 2 out]
                  }
                  frame 5 {
                    n472 = for {
                      tunnel: w1002 -> [w1005] mode=indexing
                      tunnel: bool[] [FALSE, FALSE, FALSE, FALSE, FALSE, FALSE, FALSE, FALSE, FALSE, FALSE, FALSE, FALSE, FALSE, FALSE] -> [w1004] mode=indexing
                      n473 = property class="Ctl"(reference=w1005, "Visible"=w1004) -> ()  [unwired: 1 in, 2 out]
                    }
                  }
                }
                n474 = Flatten To String(anything=w926) -> (data string=w927:string, error out=w928:errorcluster)  [unwired: 3 in, 1 out]
                n475 = call-poly <vilib>:"NI VeriStand - Set Item Property.vi"("error in (no error)"=w928, "Value"=w927, "Property Name"="Par", "Item Ref in"=w930) -> ("error out"=w931:errorcluster)  [unwired: 5 in, 2 out]
              }
              frame Error {
                n476 = call <vilib>:"Clear Errors.vi"("error in (no error)"=w1007) -> ("error out"=w1006:errorcluster)  [unwired: 5 in, 1 out]
              }
            }
          }
          event "Import 3": Value Change {
            n477 = event-data() -> ()  [unwired: 7 out]
            n478 = Unbundle By Name(w1014) -> ("O2Sensor3.Lambda Type"=w1013:T3)
            n479 = Open/Create/Replace File(error in=w1009, operation (0:open)=T16."open", access (0:read/write)=enum16{"read/write", "read-only", "write-only"}."read-only") -> (refnum out=w1012:refnum<file>, error out=w1008:errorcluster)  [unwired: 3 in, 1 out]
            n480 = case shown="No Error" w1008 {
              selector: w1008 -> [w1030 w1130]
              tunnel: [w1054 w1129] -> w1016
              tunnel: w1015 -> [w1053 _]
              tunnel: w1014 -> [w1049 _]
              tunnel: w1013 -> [w1019 _]
              tunnel: w1012 -> [w1046 _]
              frame No Error {
                w1028 = 20 ("index")
                n481 = Read from Text File(file (use dialog)=w1046, error in=w1030) -> (refnum out=w1047:refnum<file>, text=w1045:string, error out=w1048:errorcluster)  [unwired: 2 in, 1 out]
                n482 = Spreadsheet String To Array(delimiter (Tab)=",", format string="%s", spreadsheet string=w1045) -> (array=w1037:dbl[][])  [unwired: 1 in]
                n483 = Close File(refnum=w1047, error in=w1048) -> ()  [unwired: 2 out]
                n484 = Delete From Array(array=w1037, length=1, index (row)=0) -> (array with subset deleted=w1039:dbl[][])  [unwired: 1 in, 1 out]
                n485 = Index Array(array=w1039, index (col) #1=0 ("disabled index (col)"), index (col) #2=1 ("index (col)")) -> (element #1=w1040:dbl[], element #2=w1041:dbl[], element #3=w1034:dbl[], element #4=w1035:dbl[])  [unwired: 6 in]
                n486 = Build Array(w1035, w1034) -> (w1036:dbl[][])
                n487 = Build Array(w1041, w1040) -> (w1042:dbl[][])
                n488 = Transpose 2D Array(2D array=w1036) -> (transposed array=w1017:dbl[][])
                n489 = Transpose 2D Array(2D array=w1042) -> (transposed array=w1018:dbl[][])
                n490 = local read "RefArray"() -> (w1026:refnum<vi>[])
                n491 = Add(x=w1028, y=5) -> (x+y=w1027:i32)
                n492 = Array Subset(array=w1026, index=48, length=4) -> (w1021:refnum<vi>[])
                n493 = Array Subset(array=w1026, index=w1028, length=10 ("index")) -> (w1020:refnum<vi>[])
                n494 = Build Array (concatenate)(w1020, w1021) -> (w1022:refnum<vi>[])
                n495 = case shown="1" w1019 {
                  tunnel: w1022 -> [w1066 w1079 w1093 w1107 w1121 w1125]
                  tunnel: w1026 -> [w1064 w1073 w1087 w1101 w1115 _]
                  tunnel: w1028 -> [w1061 w1072 w1086 w1100 w1114 _]
                  tunnel: w1027 -> [w1059 w1071 w1085 w1099 w1113 _]
                  tunnel: w1018 -> [w1056 w1070 w1084 w1098 w1112 _]
                  tunnel: w1017 -> [w1055 w1069 w1083 w1097 w1111 _]
                  frame 0, Default {
                    w1060 = 0 ("y")
                    n496 = Add(x=w1059, y=w1060) -> (x+y=w1057:i32)
                    n497 = Add(x=w1061, y=w1060) -> (x+y=w1058:i32)
                    n498 = for {
                      tunnel: w1066 -> [w1068] mode=indexing
                      tunnel: bool[] [TRUE, FALSE, FALSE, FALSE, FALSE, TRUE, FALSE, FALSE, FALSE, FALSE, TRUE, TRUE, TRUE, TRUE] -> [w1067] mode=indexing
                      n499 = property class="Ctl"(reference=w1068, "Visible"=w1067) -> ()  [unwired: 1 in, 2 out]
                    }
                    n500 = Index Array(array=w1064, index #1=w1058, index #2=w1057) -> (element #1=w1063:refnum<vi>, element #2=w1062:refnum<vi>)
                    n501 = property class="Ctl"(reference=w1062, "Val(Sgnl)"=w1055) -> ()  [unwired: 1 in, 2 out]
                    n502 = property class="Ctl"(reference=w1063, "Val(Sgnl)"=w1056) -> ()  [unwired: 1 in, 2 out]
                  }
                  frame 1 {
                    w1076 = 1 ("y")
                    n503 = Add(x=w1071, y=w1076) -> (x+y=w1074:i32)
                    n504 = Add(x=w1072, y=w1076) -> (x+y=w1075:i32)
                    n505 = Index Array(array=w1073, index #1=w1075, index #2=w1074) -> (element #1=w1078:refnum<vi>, element #2=w1077:refnum<vi>)
                    n506 = for {
                      tunnel: w1079 -> [w1082] mode=indexing
                      tunnel: bool[] [FALSE, TRUE, FALSE, FALSE, FALSE, FALSE, TRUE, FALSE, FALSE, FALSE, TRUE, TRUE, TRUE, TRUE] -> [w1081] mode=indexing
                      n507 = property class="Ctl"(reference=w1082, "Visible"=w1081) -> ()  [unwired: 1 in, 2 out]
                    }
                    n508 = property class="Ctl"(reference=w1077, "Val(Sgnl)"=w1069) -> ()  [unwired: 1 in, 2 out]
                    n509 = property class="Ctl"(reference=w1078, "Val(Sgnl)"=w1070) -> ()  [unwired: 1 in, 2 out]
                  }
                  frame 2 {
                    w1090 = 2 ("y")
                    n510 = Add(x=w1085, y=w1090) -> (x+y=w1088:i32)
                    n511 = Add(x=w1086, y=w1090) -> (x+y=w1089:i32)
                    n512 = Index Array(array=w1087, index #1=w1089, index #2=w1088) -> (element #1=w1092:refnum<vi>, element #2=w1091:refnum<vi>)
                    n513 = for {
                      tunnel: w1093 -> [w1096] mode=indexing
                      tunnel: bool[] [FALSE, FALSE, FALSE, TRUE, FALSE, FALSE, FALSE, FALSE, TRUE, FALSE, TRUE, TRUE, TRUE, TRUE] -> [w1095] mode=indexing
                      n514 = property class="Ctl"(reference=w1096, "Visible"=w1095) -> ()  [unwired: 1 in, 2 out]
                    }
                    n515 = property class="Ctl"(reference=w1091, "Val(Sgnl)"=w1083) -> ()  [unwired: 1 in, 2 out]
                    n516 = property class="Ctl"(reference=w1092, "Val(Sgnl)"=w1084) -> ()  [unwired: 1 in, 2 out]
                  }
                  frame 3 {
                    w1104 = 3 ("y")
                    n517 = Add(x=w1099, y=w1104) -> (x+y=w1102:i32)
                    n518 = Add(x=w1100, y=w1104) -> (x+y=w1103:i32)
                    n519 = Index Array(array=w1101, index #1=w1103, index #2=w1102) -> (element #1=w1106:refnum<vi>, element #2=w1105:refnum<vi>)
                    n520 = for {
                      tunnel: w1107 -> [w1110] mode=indexing
                      tunnel: bool[] [FALSE, FALSE, TRUE, FALSE, FALSE, FALSE, FALSE, TRUE, FALSE, FALSE, TRUE, TRUE, TRUE, TRUE] -> [w1109] mode=indexing
                      n521 = property class="Ctl"(reference=w1110, "Visible"=w1109) -> ()  [unwired: 1 in, 2 out]
                    }
                    n522 = property class="Ctl"(reference=w1105, "Val(Sgnl)"=w1097) -> ()  [unwired: 1 in, 2 out]
                    n523 = property class="Ctl"(reference=w1106, "Val(Sgnl)"=w1098) -> ()  [unwired: 1 in, 2 out]
                  }
                  frame 4 {
                    w1116 = 4 ("y")
                    n524 = Add(x=w1113, y=w1116) -> (x+y=w1117:i32)
                    n525 = Add(x=w1114, y=w1116) -> (x+y=w1118:i32)
                    n526 = Index Array(array=w1115, index #1=w1118, index #2=w1117) -> (element #1=w1120:refnum<vi>, element #2=w1119:refnum<vi>)
                    n527 = for {
                      tunnel: w1121 -> [w1124] mode=indexing
                      tunnel: bool[] [FALSE, FALSE, FALSE, FALSE, TRUE, FALSE, FALSE, FALSE, FALSE, TRUE, TRUE, TRUE, TRUE, TRUE] -> [w1123] mode=indexing
                      n528 = property class="Ctl"(reference=w1124, "Visible"=w1123) -> ()  [unwired: 1 in, 2 out]
                    }
                    n529 = property class="Ctl"(reference=w1119, "Val(Sgnl)"=w1111) -> ()  [unwired: 1 in, 2 out]
                    n530 = property class="Ctl"(reference=w1120, "Val(Sgnl)"=w1112) -> ()  [unwired: 1 in, 2 out]
                  }
                  frame 5 {
                    n531 = for {
                      tunnel: w1125 -> [w1128] mode=indexing
                      tunnel: bool[] [FALSE, FALSE, FALSE, FALSE, FALSE, FALSE, FALSE, FALSE, FALSE, FALSE, FALSE, FALSE, FALSE, FALSE] -> [w1127] mode=indexing
                      n532 = property class="Ctl"(reference=w1128, "Visible"=w1127) -> ()  [unwired: 1 in, 2 out]
                    }
                  }
                }
                n533 = Flatten To String(anything=w1049) -> (data string=w1050:string, error out=w1051:errorcluster)  [unwired: 3 in, 1 out]
                n534 = call-poly <vilib>:"NI VeriStand - Set Item Property.vi"("error in (no error)"=w1051, "Value"=w1050, "Property Name"="Par", "Item Ref in"=w1053) -> ("error out"=w1054:errorcluster)  [unwired: 5 in, 2 out]
              }
              frame Error {
                n535 = call <vilib>:"Clear Errors.vi"("error in (no error)"=w1130) -> ("error out"=w1129:errorcluster)  [unwired: 5 in, 1 out]
              }
            }
          }
          event "Import 4": Value Change {
            n536 = event-data() -> ()  [unwired: 7 out]
            n537 = Unbundle By Name(w1137) -> ("O2Sensor4.Lambda Type"=w1136:T3)
            n538 = Open/Create/Replace File(error in=w1132, operation (0:open)=T16."open", access (0:read/write)=enum16{"read/write", "read-only", "write-only"}."read-only") -> (refnum out=w1135:refnum<file>, error out=w1131:errorcluster)  [unwired: 3 in, 1 out]
            n539 = case shown="No Error" w1131 {
              selector: w1131 -> [w1153 w1253]
              tunnel: [w1177 w1252] -> w1139
              tunnel: w1138 -> [w1176 _]
              tunnel: w1137 -> [w1172 _]
              tunnel: w1136 -> [w1142 _]
              tunnel: w1135 -> [w1169 _]
              frame No Error {
                w1151 = 30 ("index")
                n540 = Read from Text File(file (use dialog)=w1169, error in=w1153) -> (refnum out=w1170:refnum<file>, text=w1168:string, error out=w1171:errorcluster)  [unwired: 2 in, 1 out]
                n541 = Spreadsheet String To Array(delimiter (Tab)=",", format string="%s", spreadsheet string=w1168) -> (array=w1160:dbl[][])  [unwired: 1 in]
                n542 = Close File(refnum=w1170, error in=w1171) -> ()  [unwired: 2 out]
                n543 = Delete From Array(array=w1160, length=1, index (row)=0) -> (array with subset deleted=w1162:dbl[][])  [unwired: 1 in, 1 out]
                n544 = Index Array(array=w1162, index (col) #1=0 ("disabled index (col)"), index (col) #2=1 ("index (col)")) -> (element #1=w1163:dbl[], element #2=w1164:dbl[], element #3=w1157:dbl[], element #4=w1158:dbl[])  [unwired: 6 in]
                n545 = Build Array(w1158, w1157) -> (w1159:dbl[][])
                n546 = Build Array(w1164, w1163) -> (w1165:dbl[][])
                n547 = Transpose 2D Array(2D array=w1159) -> (transposed array=w1140:dbl[][])
                n548 = Transpose 2D Array(2D array=w1165) -> (transposed array=w1141:dbl[][])
                n549 = local read "RefArray"() -> (w1149:refnum<vi>[])
                n550 = Add(x=w1151, y=5) -> (x+y=w1150:i32)
                n551 = Array Subset(array=w1149, index=52, length=4) -> (w1144:refnum<vi>[])
                n552 = Array Subset(array=w1149, index=w1151, length=10 ("index")) -> (w1143:refnum<vi>[])
                n553 = Build Array (concatenate)(w1143, w1144) -> (w1145:refnum<vi>[])
                n554 = case shown="1" w1142 {
                  tunnel: w1145 -> [w1189 w1202 w1216 w1230 w1244 w1248]
                  tunnel: w1149 -> [w1187 w1196 w1210 w1224 w1238 _]
                  tunnel: w1151 -> [w1184 w1195 w1209 w1223 w1237 _]
                  tunnel: w1150 -> [w1182 w1194 w1208 w1222 w1236 _]
                  tunnel: w1141 -> [w1179 w1193 w1207 w1221 w1235 _]
                  tunnel: w1140 -> [w1178 w1192 w1206 w1220 w1234 _]
                  frame 0, Default {
                    w1183 = 0 ("y")
                    n555 = Add(x=w1182, y=w1183) -> (x+y=w1180:i32)
                    n556 = Add(x=w1184, y=w1183) -> (x+y=w1181:i32)
                    n557 = for {
                      tunnel: w1189 -> [w1191] mode=indexing
                      tunnel: bool[] [TRUE, FALSE, FALSE, FALSE, FALSE, TRUE, FALSE, FALSE, FALSE, FALSE, TRUE, TRUE, TRUE, TRUE] -> [w1190] mode=indexing
                      n558 = property class="Ctl"(reference=w1191, "Visible"=w1190) -> ()  [unwired: 1 in, 2 out]
                    }
                    n559 = Index Array(array=w1187, index #1=w1181, index #2=w1180) -> (element #1=w1186:refnum<vi>, element #2=w1185:refnum<vi>)
                    n560 = property class="Ctl"(reference=w1185, "Val(Sgnl)"=w1178) -> ()  [unwired: 1 in, 2 out]
                    n561 = property class="Ctl"(reference=w1186, "Val(Sgnl)"=w1179) -> ()  [unwired: 1 in, 2 out]
                  }
                  frame 1 {
                    w1199 = 1 ("y")
                    n562 = Add(x=w1194, y=w1199) -> (x+y=w1197:i32)
                    n563 = Add(x=w1195, y=w1199) -> (x+y=w1198:i32)
                    n564 = Index Array(array=w1196, index #1=w1198, index #2=w1197) -> (element #1=w1201:refnum<vi>, element #2=w1200:refnum<vi>)
                    n565 = for {
                      tunnel: w1202 -> [w1205] mode=indexing
                      tunnel: bool[] [FALSE, TRUE, FALSE, FALSE, FALSE, FALSE, TRUE, FALSE, FALSE, FALSE, TRUE, TRUE, TRUE, TRUE] -> [w1204] mode=indexing
                      n566 = property class="Ctl"(reference=w1205, "Visible"=w1204) -> ()  [unwired: 1 in, 2 out]
                    }
                    n567 = property class="Ctl"(reference=w1200, "Val(Sgnl)"=w1192) -> ()  [unwired: 1 in, 2 out]
                    n568 = property class="Ctl"(reference=w1201, "Val(Sgnl)"=w1193) -> ()  [unwired: 1 in, 2 out]
                  }
                  frame 2 {
                    w1213 = 2 ("y")
                    n569 = Add(x=w1208, y=w1213) -> (x+y=w1211:i32)
                    n570 = Add(x=w1209, y=w1213) -> (x+y=w1212:i32)
                    n571 = Index Array(array=w1210, index #1=w1212, index #2=w1211) -> (element #1=w1215:refnum<vi>, element #2=w1214:refnum<vi>)
                    n572 = for {
                      tunnel: w1216 -> [w1219] mode=indexing
                      tunnel: bool[] [FALSE, FALSE, FALSE, TRUE, FALSE, FALSE, FALSE, FALSE, TRUE, FALSE, TRUE, TRUE, TRUE, TRUE] -> [w1218] mode=indexing
                      n573 = property class="Ctl"(reference=w1219, "Visible"=w1218) -> ()  [unwired: 1 in, 2 out]
                    }
                    n574 = property class="Ctl"(reference=w1214, "Val(Sgnl)"=w1206) -> ()  [unwired: 1 in, 2 out]
                    n575 = property class="Ctl"(reference=w1215, "Val(Sgnl)"=w1207) -> ()  [unwired: 1 in, 2 out]
                  }
                  frame 3 {
                    w1227 = 3 ("y")
                    n576 = Add(x=w1222, y=w1227) -> (x+y=w1225:i32)
                    n577 = Add(x=w1223, y=w1227) -> (x+y=w1226:i32)
                    n578 = Index Array(array=w1224, index #1=w1226, index #2=w1225) -> (element #1=w1229:refnum<vi>, element #2=w1228:refnum<vi>)
                    n579 = for {
                      tunnel: w1230 -> [w1233] mode=indexing
                      tunnel: bool[] [FALSE, FALSE, TRUE, FALSE, FALSE, FALSE, FALSE, TRUE, FALSE, FALSE, TRUE, TRUE, TRUE, TRUE] -> [w1232] mode=indexing
                      n580 = property class="Ctl"(reference=w1233, "Visible"=w1232) -> ()  [unwired: 1 in, 2 out]
                    }
                    n581 = property class="Ctl"(reference=w1228, "Val(Sgnl)"=w1220) -> ()  [unwired: 1 in, 2 out]
                    n582 = property class="Ctl"(reference=w1229, "Val(Sgnl)"=w1221) -> ()  [unwired: 1 in, 2 out]
                  }
                  frame 4 {
                    w1239 = 4 ("y")
                    n583 = Add(x=w1236, y=w1239) -> (x+y=w1240:i32)
                    n584 = Add(x=w1237, y=w1239) -> (x+y=w1241:i32)
                    n585 = Index Array(array=w1238, index #1=w1241, index #2=w1240) -> (element #1=w1243:refnum<vi>, element #2=w1242:refnum<vi>)
                    n586 = for {
                      tunnel: w1244 -> [w1247] mode=indexing
                      tunnel: bool[] [FALSE, FALSE, FALSE, FALSE, TRUE, FALSE, FALSE, FALSE, FALSE, TRUE, TRUE, TRUE, TRUE, TRUE] -> [w1246] mode=indexing
                      n587 = property class="Ctl"(reference=w1247, "Visible"=w1246) -> ()  [unwired: 1 in, 2 out]
                    }
                    n588 = property class="Ctl"(reference=w1242, "Val(Sgnl)"=w1234) -> ()  [unwired: 1 in, 2 out]
                    n589 = property class="Ctl"(reference=w1243, "Val(Sgnl)"=w1235) -> ()  [unwired: 1 in, 2 out]
                  }
                  frame 5 {
                    n590 = for {
                      tunnel: w1248 -> [w1251] mode=indexing
                      tunnel: bool[] [FALSE, FALSE, FALSE, FALSE, FALSE, FALSE, FALSE, FALSE, FALSE, FALSE, FALSE, FALSE, FALSE, FALSE] -> [w1250] mode=indexing
                      n591 = property class="Ctl"(reference=w1251, "Visible"=w1250) -> ()  [unwired: 1 in, 2 out]
                    }
                  }
                }
                n592 = Flatten To String(anything=w1172) -> (data string=w1173:string, error out=w1174:errorcluster)  [unwired: 3 in, 1 out]
                n593 = call-poly <vilib>:"NI VeriStand - Set Item Property.vi"("error in (no error)"=w1174, "Value"=w1173, "Property Name"="Par", "Item Ref in"=w1176) -> ("error out"=w1177:errorcluster)  [unwired: 5 in, 2 out]
              }
              frame Error {
                n594 = call <vilib>:"Clear Errors.vi"("error in (no error)"=w1253) -> ("error out"=w1252:errorcluster)  [unwired: 5 in, 1 out]
              }
            }
          }
          event "Manual": Value Change {
            w1257 = T18 6 items=["User Home"=0, "User Desktop"=1, "User Documents"=2, "User Application Data"=3, "User Preferences"=4, "User Temporary"=5, "Public Documents"=6, "Public Application Data"=7, "Public Preferences"=8, "Public Cache"=13, "System Core Libraries"=9, "System Installed Libraries"=10, "Application Files"=11, "Boot Volume Root"=12] ("system directory type")
            n595 = event-data() -> ()  [unwired: 2 out]
            n596 = call <vilib>:"Get System Directory.vi"("system directory type"=w1257) -> ("system directory"=w1258:path)  [unwired: 10 in]
            n597 = Build Path(base path=w1258, name or relative path=path "National Instruments/NI VeriStand 2017/Custom Devices/Alma Automotive/2Ch_O2SensorSim" ("system directory")) -> (appended path=w1260:path)
            n598 = Build Path(base path=w1260, name or relative path="Manual.pdf") -> (appended path=w1256:path)
            n599 = call <vilib>:"Open Acrobat Document.vi"("error in (no error)"=w1255, "acrobat document"=w1256) -> ("error out"=w1254:errorcluster)  [unwired: 5 in]
          }
        }
        n600 = call-poly <userlib>:"Data Changed__ogtk.vi"("Variant"=w527) -> ("Changed"=w504:bool)
        n601 = Or(x=w504, y=w531) -> (x .or. y?=w500:bool)
        n602 = Or(x=w502, y=w500) -> (x .or. y?=w501:bool)
        n603 = case shown="True" w501 {
          tunnel: w505 -> [_ w543]
          tunnel: w503 -> [_ w542]
          frame False {
          }
          frame True {
            n604 = Index Array(array=w543, index=w542) -> (element=w550:T14)
            n605 = Unbundle By Name(w550) -> ("Lambda Type"=w551:T3)
            n606 = case shown="4" w551 {
              tunnel: w550 -> [w556 w561 w566 w571 w576]
              tunnel: [w555 w560 w565 w570 w575] -> w549
              tunnel: [w554 w559 w564 w569 w574] -> w548
              tunnel: [w553 w558 w563 w568 w573] -> w546
              tunnel: [w552 w557 w562 w567 w572] -> w545
              frame 0, Default {
                n607 = Unbundle By Name(w556) -> ("Lambda.LSU4.2 Lambda"=w555:dbl[], "Lambda.LSU4.2 Ip"=w554:dbl[], "Temp.LSU4.2 Temp"=w553:dbl[], "Temp.LSU4.2 Ohm"=w552:dbl[])
              }
              frame 1 {
                n608 = Unbundle By Name(w561) -> ("Lambda.LSU4.9 Lambda"=w560:dbl[], "Lambda.LSU4.9 Ip"=w559:dbl[], "Temp.LSU4.9 Temp"=w558:dbl[], "Temp.LSU4.9 Ohm"=w557:dbl[])
              }
              frame 2 {
                n609 = Unbundle By Name(w566) -> ("Lambda.LZA03 Lambda"=w565:dbl[], "Lambda.LZA03 Ip"=w564:dbl[], "Temp.LZA03 Temp"=w563:dbl[], "Temp.LZA03 Ohm"=w562:dbl[])
              }
              frame 3 {
                n610 = Unbundle By Name(w571) -> ("Lambda.LZA08 Lambda"=w570:dbl[], "Lambda.LZA08 Ip"=w569:dbl[], "Temp.LZA08 Temp"=w568:dbl[], "Temp.LZA08 Ohm"=w567:dbl[])
              }
              frame 4 {
                n611 = Unbundle By Name(w576) -> ("Lambda.Custom Lambda"=w575:dbl[], "Lambda.Custom Ip"=w574:dbl[], "Temp.Custom Temp"=w573:dbl[], "Temp.Custom Ohm"=w572:dbl[])
              }
            }
            n612 = Bundle("Custom Lambda"=w549, "Custom Ip"=w548) -> (→"l VS IP [mA]":T1)  [unwired: 1 in]
            n613 = Bundle("Custom Temp"=w546, "Custom Ohm"=w545) -> (→"Temperature [°C] VS Rs [W]":cluster{"Custom Temp":dbl[], "Custom Ohm":dbl[]})  [unwired: 1 in]
          }
        }
        n614 = case shown="True" w500 {
          frame False {
          }
          frame True {
            n615 = property on="ParamUpdate" class="Bool (strict)"("Val(Sgnl)"=TRUE ("Value (Signaling)")) -> ()  [unwired: 2 in, 2 out]
          }
        }
        n616 = call <vilib>:"Simple Error Handler.vi"("error in (no error)"=w536) -> ("error out"=w535:errorcluster)  [unwired: 1 in, 7 out]
        n617 = call <vilib>:"Clear Errors.vi"("error in (no error)"=w535) -> ("error out"=w534:errorcluster)  [unwired: 1 in, 5 out]
      }
      n618 = Unregister For Events(event registration refnum=w499, error in=w498) -> (error out=w497:errorcluster)
    }
    frame Error {
      n619 = call <vilib>:"Simple Error Handler.vi"("error in (no error)"=w1264) -> ("error out"=w1263:errorcluster)  [unwired: 1 in, 7 out]
      n620 = call <vilib>:"Clear Errors.vi"("error in (no error)"=w1263) -> ("error out"=w1262:errorcluster)  [unwired: 1 in, 5 out]
    }
  }
  n621 = disable-structure shown="Enabled" {
    disable-tunnel: [w1266 w1268] -> w14
    disable-tunnel: w9 -> [w1265 w1268]
    frame Enabled {
      n622 = invoke class="VI" method="FP.Close"(error in=w1265) -> (error out=w1267:errorcluster)  [unwired: 2 in, 2 out]
      n623 = call <vilib>:"NI VeriStand - Signal When Ready for Shutdown.vi"("error in (no error)"=w1267) -> ("error out"=w1266:errorcluster)  [unwired: 10 out]
    }
    frame Disabled {
    }
  }
  "error out" <- w14
